vi "Autonomous Independent.vi"() -> ()   [LabVIEW 2015]
doc: "This VI is called when autonomous begins, and will automatically be terminated when autonomous ends. You can carry out timed or sensor driven robot movement independently without needing to return to the caller."
uses:
  <vilib>/Rock Robotics/WPI/RobotDrive/WPI_RobotDriveArcadeDrive_Standard(NoSaturation).vi
  <vilib>/Rock Robotics/Network Tables/NT Read Number.vi
  <vilib>/addons/control/pid/NI_PID_pid.lvlib
  drive/drive.lvclass
  <vilib>/Rock Robotics/Network Tables/NT Write Number.vi
  <vilib>/Rock Robotics/Network Tables/NT Read Boolean.vi
  Robot Global Data.vi
  <vilib>/addons/control/pid/pid.llb/PID (DBL).vi
  <vilib>/Rock Robotics/Network Tables/NT Write Boolean.vi
panel:
  in  "PID turn angle gains":T1={"proportional gain (Kc)"=0.07, "integral time (Ti, min)"=0.0, "derivative time (Td, min)"=1e-05}
  in  "PID arm gains":T1={"proportional gain (Kc)"=1.1, "integral time (Ti, min)"=0.008, "derivative time (Td, min)"=0.0001}
  in  "PID control on":bool
  in  "Angle A?":bool=TRUE
  in  "angle A 2":dbl=30.0
  in  "angle B 2":dbl=90.0
  out "Waveform Chart arm":cluster{"angle B 2":dbl, "Arm Angle":dbl, dbl}(graph)
  in  "Chart slowing 2":i32(knob)=3 scale=1.0..10.0
  in  "Shooter control":dbl(slide) scale=-1.0..1.0
  in  "Arm control":dbl(slide) scale=-1.0..1.0
  in  "Chart slowing":i32(knob)=1 scale=1.0..10.0
  in  "angle B":dbl=90.0
  in  "angle A":dbl
  in  "Reset Gyro":bool
  out "Waveform Chart":cluster{"f":dbl, dbl}(graph)
  in  "Which angle?":bool=TRUE
  out "Stop Wheel Loop":bool
  # "Be sure to right-click and choose Data Operations>>Make Current Value default if you want to save the array values with the VI"
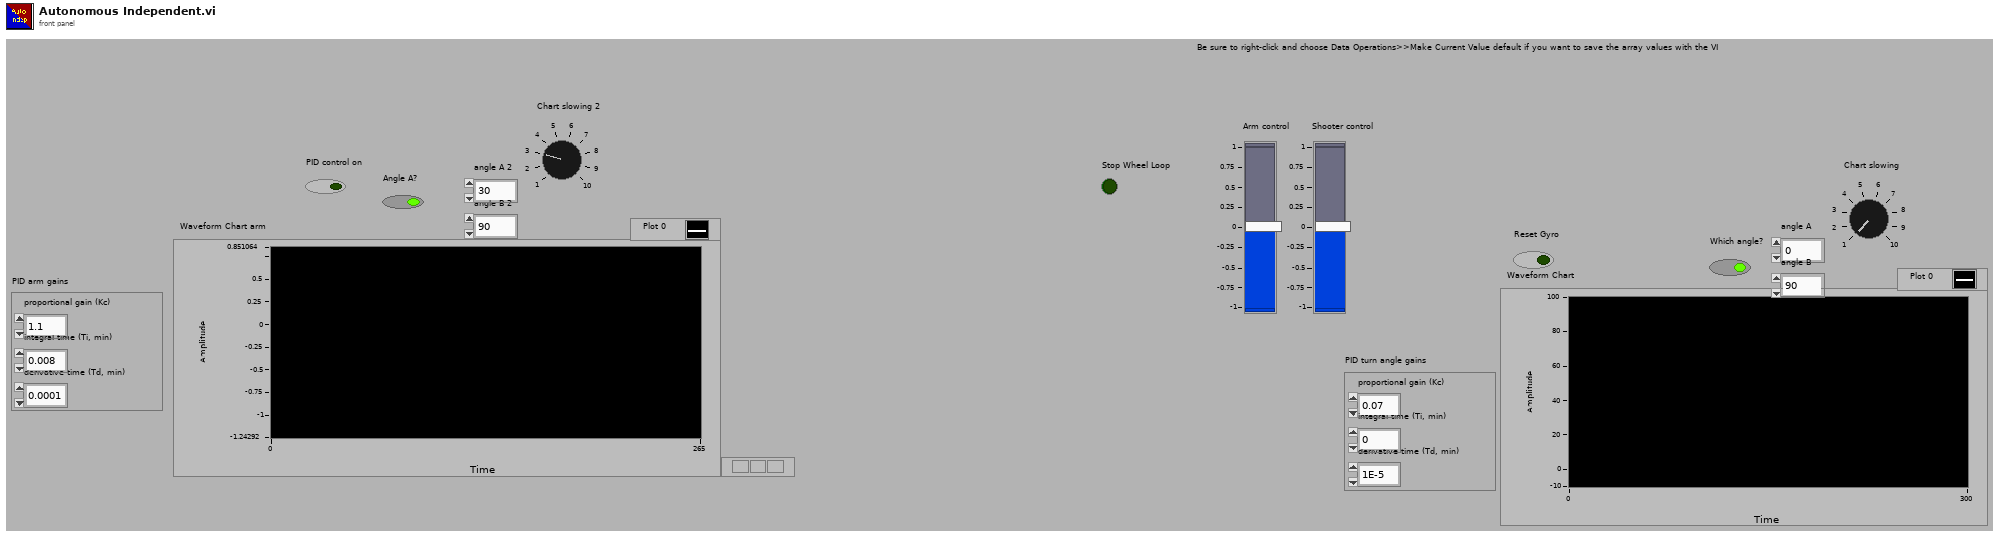
[diagram p1: front panel]
types:
  T1 = cluster{"proportional gain (Kc)":dbl, "integral time (Ti, min)":dbl, "derivative time (Td, min)":dbl}
  T2 = typedef "WPI_GyroDevRef.ctl" = cluster{"DevStatus":errorcluster, "Analog Channel":T3, "Offset":dbl, "Gain (VoltsPerDegree/Second)":dbl, "Gyro Type":enum16{"Analog", "XRS450"}, "Handle":i32, "SPI Bus":T4, "Device Found":bool, "Sample Rate":dbl, "Calibrate On Open":bool}
  T3 = typedef "FPGA_AIChannel.ctl" = enum8{"AI 0", "AI 1", "AI 2", "AI 3", "AI MXP 0", "AI MXP 1", "AI MXP 2", "AI MXP 3", "Invalid"}
  T4 = typedef "spi_bus.ctl" = enum16{"SPI On-Board, CS0", "SPI On-Board, CS1", "SPI On-Board, CS2", "SPI On-Board, CS3", "SPI MXP", "Invalid"}
  T5 = typedef "WPI_PotentiometerDevRef.ctl" = cluster{"DevStatus":errorcluster, "Analog Channel":T3, "Invert Output":bool}
  T6 = typedef "WPI_RobotDriveDevRef.ctl" = cluster{"DevStatus":errorcluster, "Motors[]":T7[], "Square Inputs":bool, "Max Output":dbl}
  T7 = typedef "WPI_MotorControlDeviceRef.ctl" = cluster{"DeviceStatus":errorcluster, "Type":T8, "PWM":cluster{"PWM Channel":T9, "DeadBand":T10}, "CAN":cluster{"Device Number":u8, "Control Mode":T11, "Semaphore":T12, "Max Vout":dbl, "TalonSRX Control Mode":T13}, "Invert":bool}
  T8 = typedef "WPI_MotorControlType.ctl" = enum16{"PWM", "CAN", "CANTalonSRX"}
  T9 = typedef "FPGA_DIOPWMChannel.ctl" = enum8{"PWM 0", "PWM 1", "PWM 2", "PWM 3", "PWM 4", "PWM 5", "PWM 6", "PWM 7", "PWM 8", "PWM 9", "PWM MXP 0", "PWM MXP 1", "PWM MXP 2", "PWM MXP 3", "PWM MXP 4", "PWM MXP 5", "PWM MXP 6", "PWM MXP 7", "PWM MXP 8", "PWM MXP 9", "Invalid"}
  T10 = typedef "WPI_PWMDeadband.ctl" = cluster{"Name":string, "maxPositivePwm":i32, "minPositivePwm":i32, "centerPwm":i32, "maxNegativePwm":i32, "minNegativePwm":i32, "angularRange":u16}
  T11 = typedef "WPI_CANJaguar_ControlMode.ctl" = enum8{"Percent VBus", "Current", "Speed", "Position", "Voltage"}
  T12 = typedef "Semaphore RefNum" = refnum<k1>
  T13 = typedef "WPI_CANTalonSRX_APIControlMode.ctl" = enum8{"Percent VBus", "Speed", "Position", "Slave", "Unchanged / Invalid", "Voltage Compensation", "Current", "Motion Profile"}
  T14 = typedef "WPI_SwitchDevRef.ctl" = cluster{"DevStatus":errorcluster, "DIO Channel":T15, "CntIndex":T16, "Normally Closed":bool}
  T15 = typedef "FPGA_DIOChannel.ctl" = enum8{"DIO 0", "DIO 1", "DIO 2", "DIO 3", "DIO 4", "DIO 5", "DIO 6", "DIO 7", "DIO 8", "DIO 9", "DIO MXP 0", "DIO MXP 1", "DIO MXP 2", "DIO MXP 3", "DIO MXP 4", "DIO MXP 5", "DIO MXP 6", "DIO MXP 7", "DIO MXP 8", "DIO MXP 9", "DIO MXP 10", "DIO MXP 11", "DIO MXP 12", "DIO MXP 13", "DIO MXP 14", "DIO MXP 15", "Invalid"}
  T16 = typedef "FPGA_CounterCtrSystemIndex.ctl" = enum8{"Ctr 0", "Ctr 1", "Ctr 2", "Ctr 3", "Ctr 4", "Ctr 5", "Ctr 6", "Ctr 7", "Invalid"}
  T17 = typedef "WPI_AccelerometerDevRef.ctl" = cluster{"DevStatus":errorcluster, "Scaling":T18, "Analog Channels":T19, "I2C Bus":T20, "SPI Bus":T4, "Accel Range":T21, "ADXL Axes":T22, "Handle":i32, "Device Address":u8, "Accel Type":enum16{"Analog", "ADXL345 I2C", "ADXL345 SPI", "Internal", "ADXL362 SPI"}}
  T18 = typedef "WPI_AccelerometerScaling.ctl" = cluster{"Gain (VoltsPerG)":dbl, "Center Voltage":dbl}
  T19 = typedef "WPI_AccelerometerAnalogChannels.ctl" = cluster{"X-Axis":T3, "Y-Axis":T3, "Z-Axis":T3}
  T20 = typedef "i2c_bus.ctl" = enum16{"I2C On-Board", "I2C MXP", "Invalid"}
  T21 = typedef "ADXL345 Range.ctl" = u8
  T22 = typedef "WPI_AccelerometerADXL345 Axes.ctl" = cluster{"X-Axis":bool, "Y-Axis":bool, "Z-Axis":bool}
  T23 = cluster{"X-Axis":dbl, "Y-Axis":dbl, "Z-Axis":dbl}
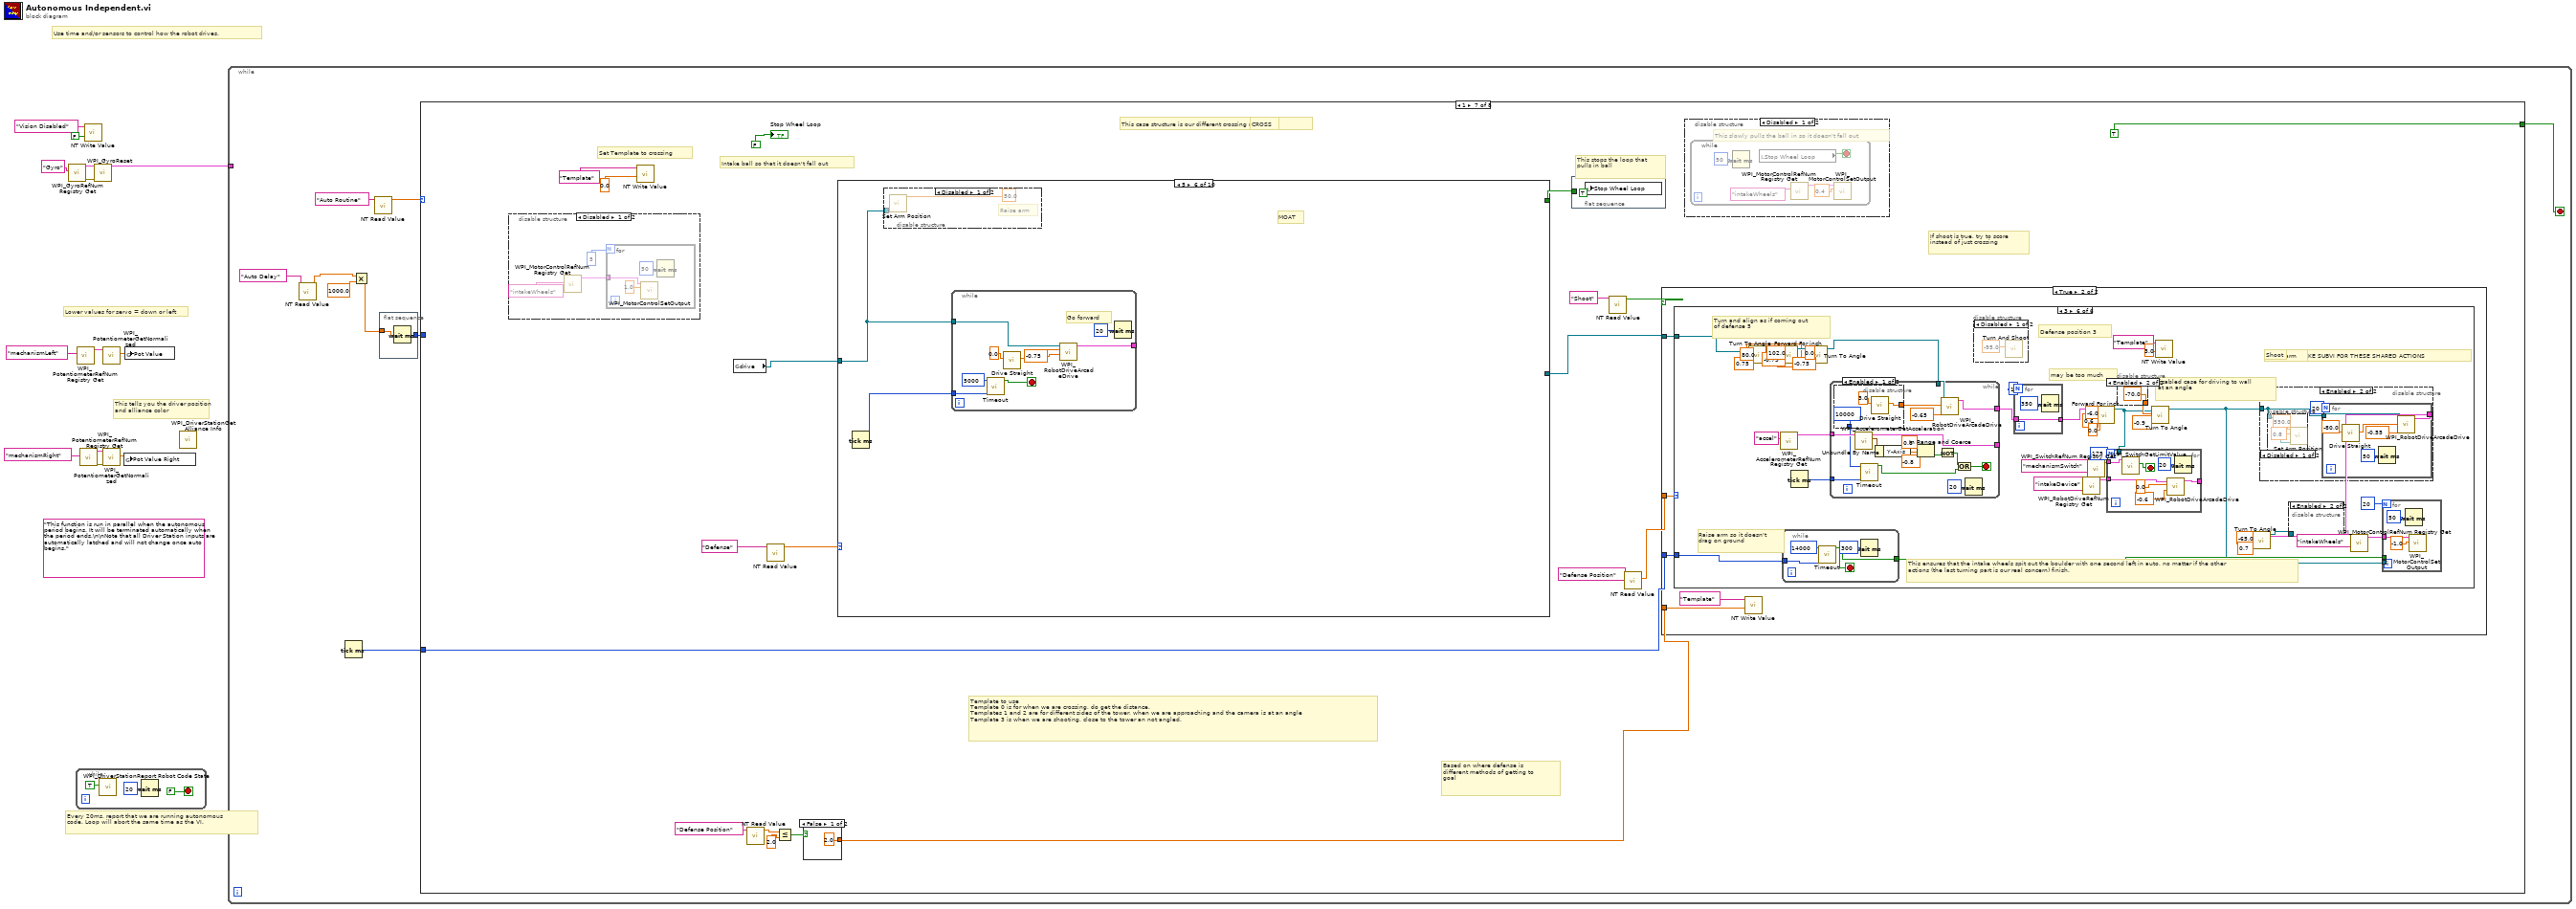
[diagram p0: block diagram]
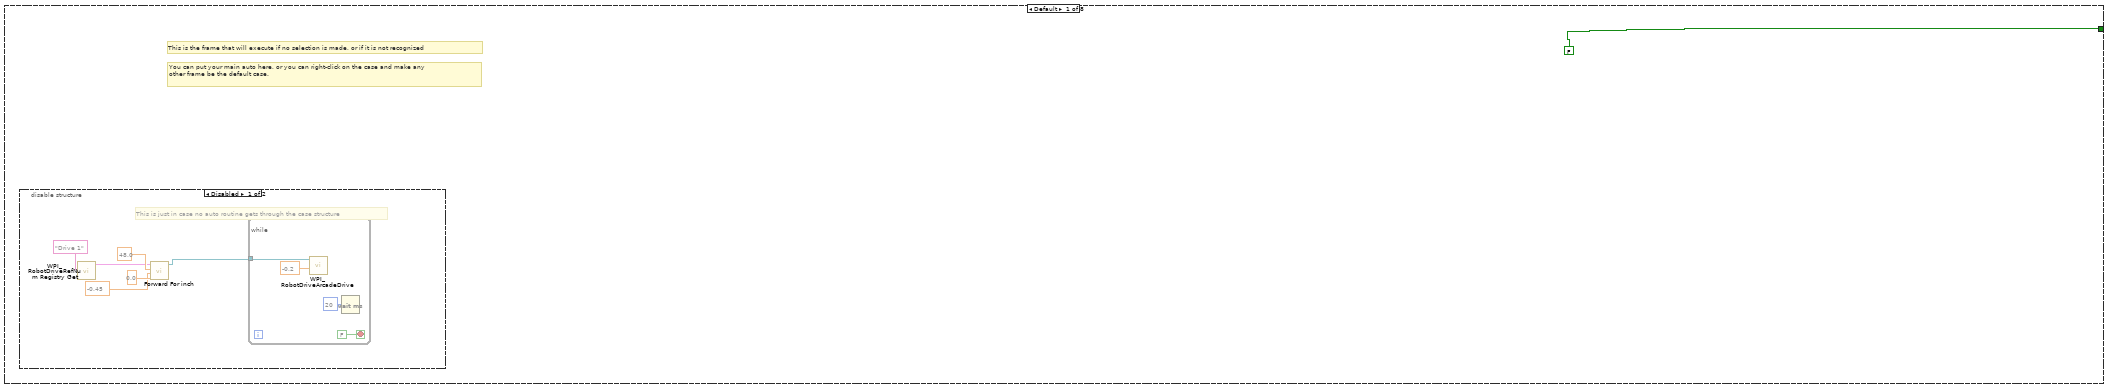
[diagram p2: hidden frame]
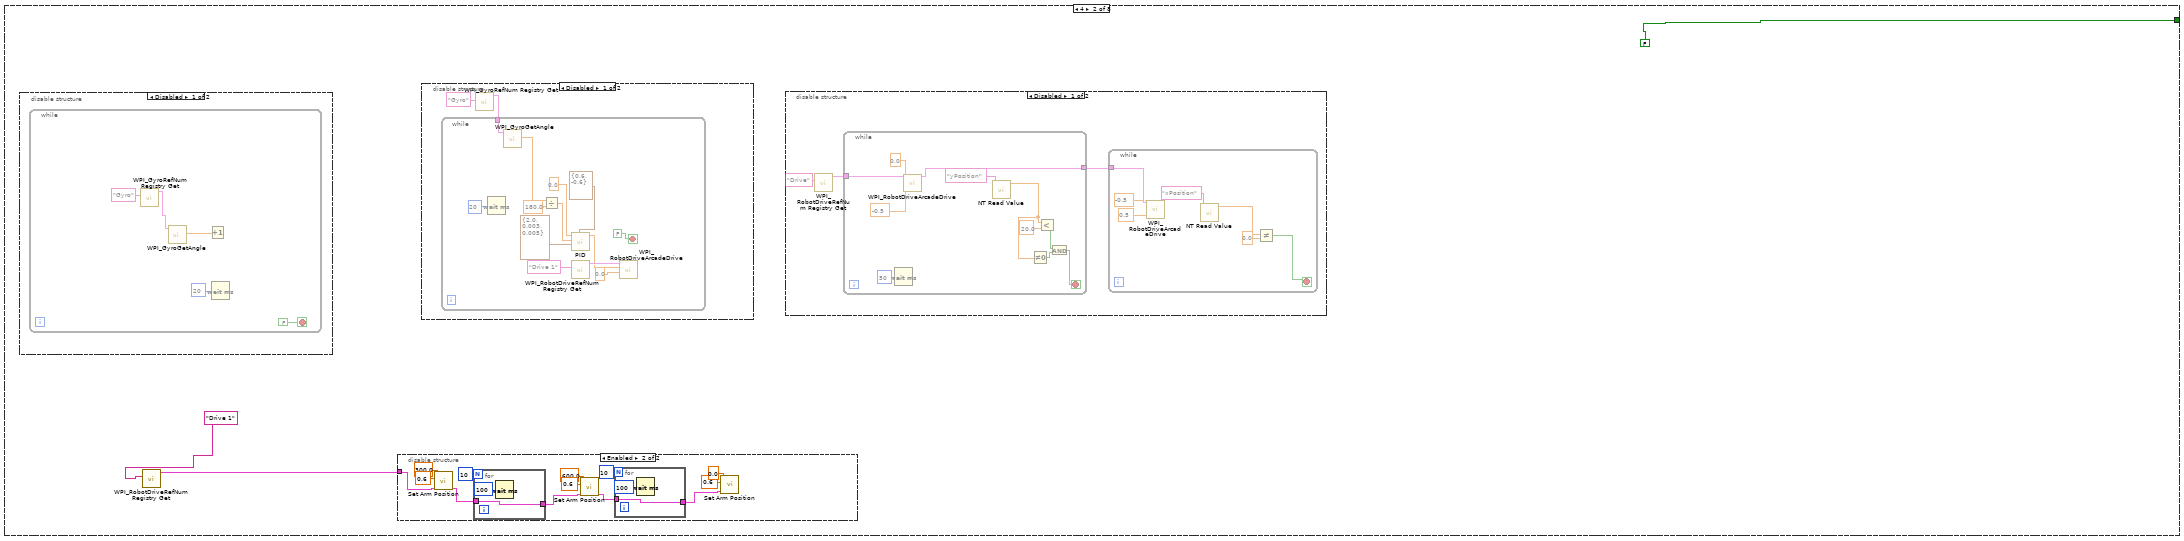
[diagram p4: hidden frame]
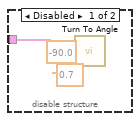
[diagram p5: hidden frame]
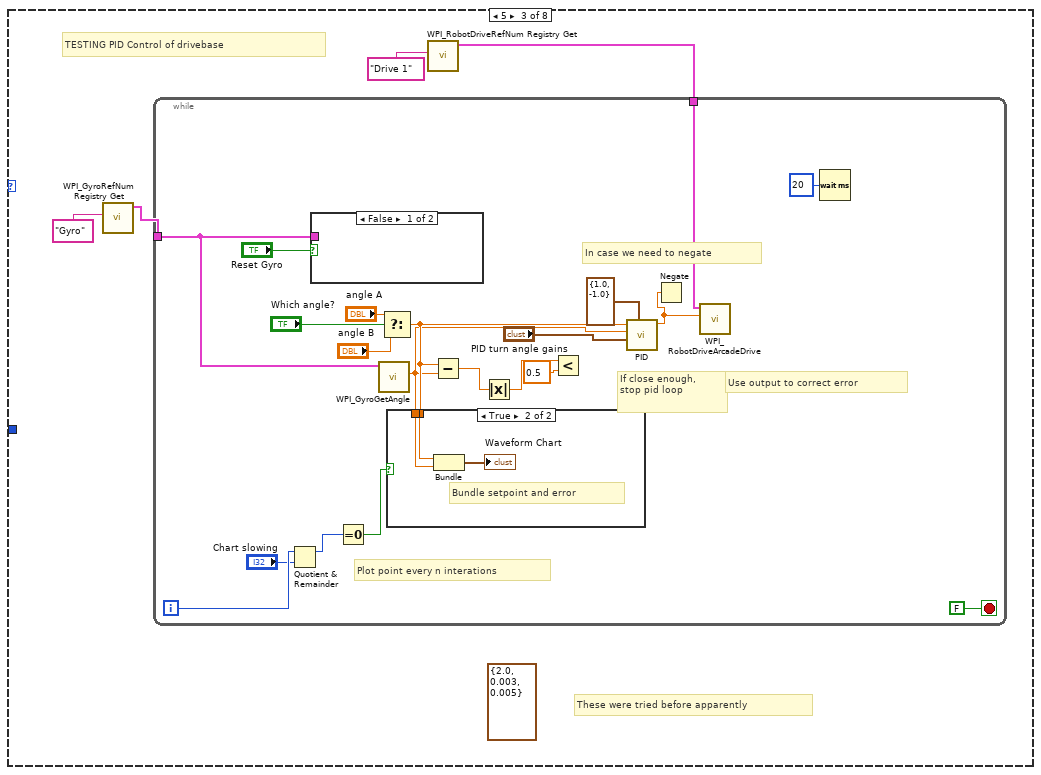
[diagram p9: hidden frame]
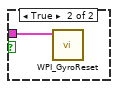
[diagram p11: hidden frame]
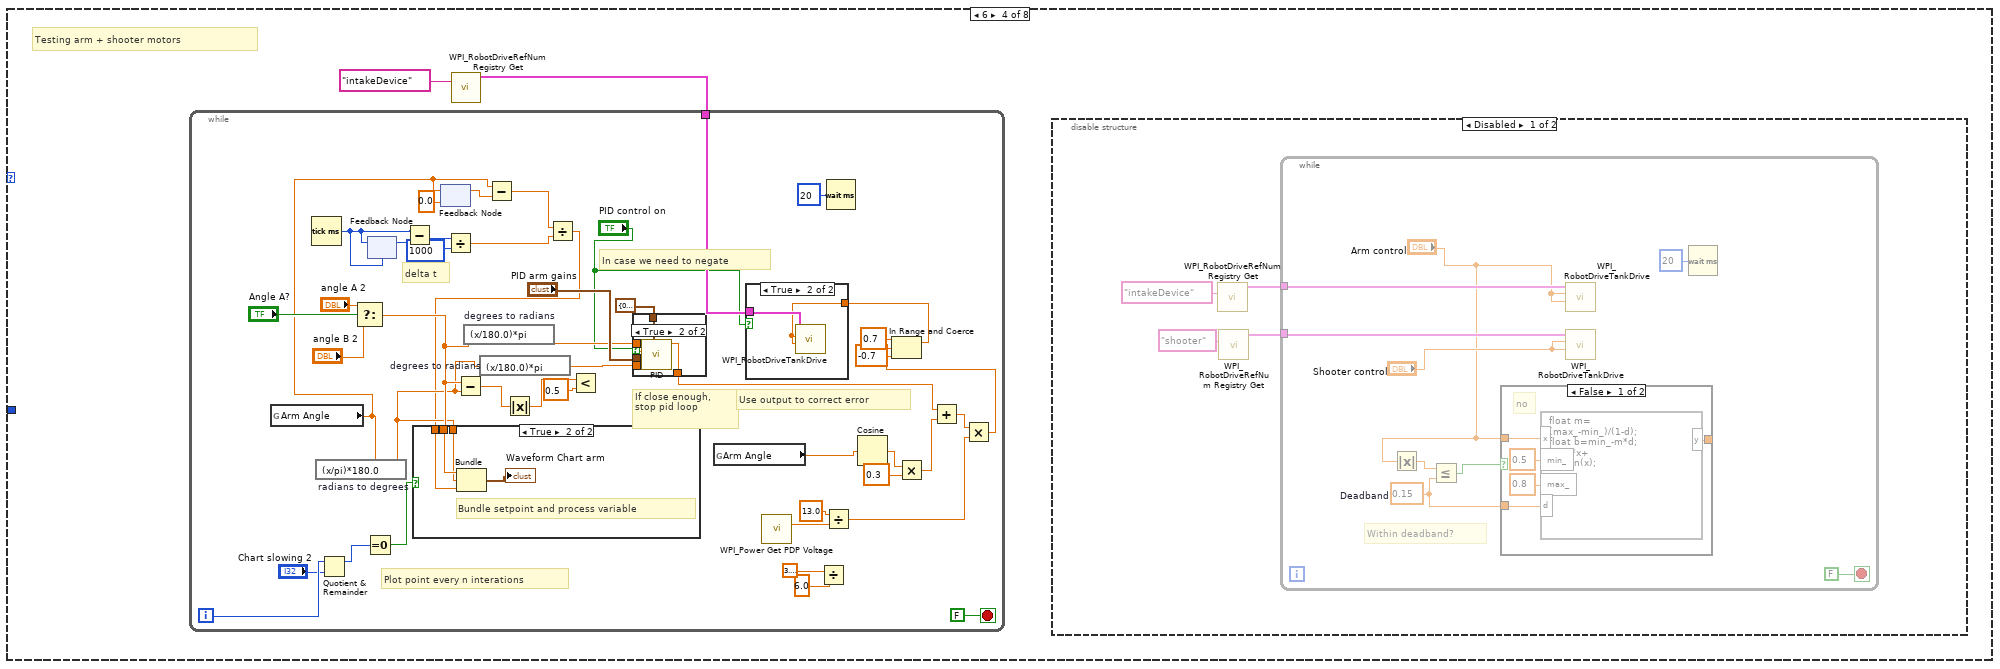
[diagram p12: hidden frame]
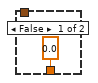
[diagram p14: hidden frame]
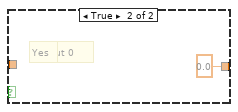
[diagram p16: hidden frame]
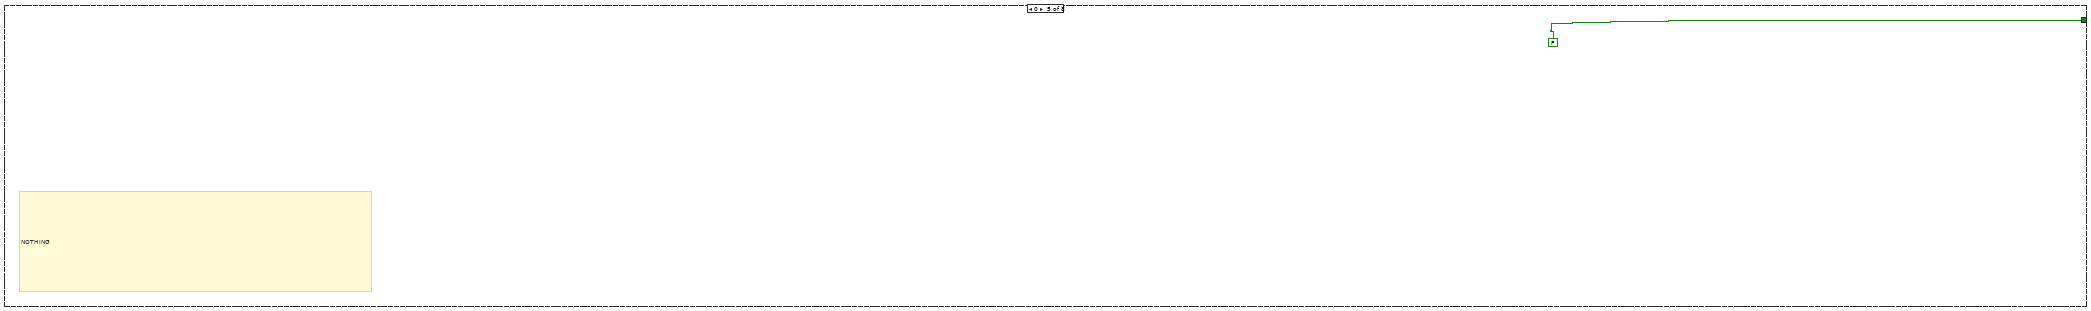
[diagram p18: hidden frame]
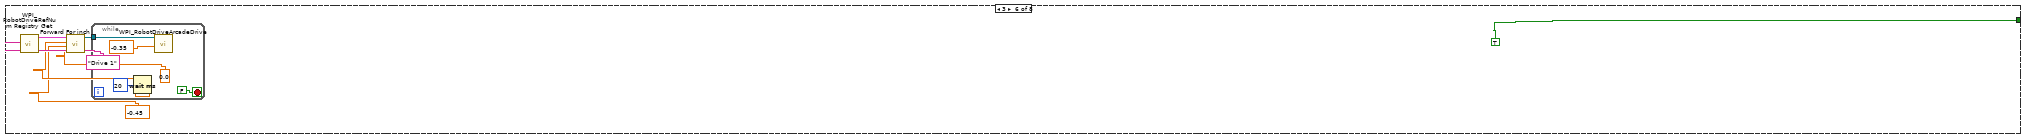
[diagram p19: hidden frame]
diagram:
  (unwired) "This function is run in parallel when the autonomous period begins. It will be terminated automatically when the period ends.\n\nNote that all Driver Station inputs are automatically latched and will not change once auto begins."
  # "Lower values for servo = down or left"
  # "Use time and/or sensors to control how the robot drives."
  # "Every 20ms, report that we are running autonomous\ncode. Loop will abort the same time as the VI."
  # "This tells you the driver position\nand alliance color"
  n1 = call <vilib>:"WPI_GyroRefNum Registry Get.vi"("refnum name"="Gyro") -> ("error out"=w13:errorcluster, "GyroDevRef"=w12:T2)  [unwired: 9 in]
  n2 = while {
    stop <- FALSE stop-if-true
    n3 = call <vilib>:"WPI_DriverStationReport Robot Code State.vi"("Autonomous"=TRUE) -> ()  [unwired: 10 in, 1 out]
    n4 = Wait (ms)(milliseconds to wait=u32 20) -> ()  [unwired: 1 out]
  }
  n5 = call <vilib>:"WPI_PotentiometerRefNum Registry Get.vi"("refnum name"="mechanismLeft") -> ("PotDevRef"=w5:T5)  [unwired: 9 in, 1 out]
  n6 = call <vilib>:"WPI_PotentiometerRefNum Registry Get.vi"("refnum name"="mechanismRight") -> ("error out"=w4:errorcluster, "PotDevRef"=w3:T5)  [unwired: 9 in]
  n7 = call-poly <vilib>:"NT Write Value.vi"("Boolean"=FALSE, "Name"="Vision Disabled") -> ()  [unwired: 9 in, 1 out]
  n8 = call <vilib>:"WPI_GyroReset.vi"("error in"=w13, "GyroDevRef"=w12) -> ("GyroDevRef"=w1:T2)  [unwired: 8 in, 1 out]
  n9 = call <vilib>:"WPI_PotentiometerGetNormalized.vi"("PotDevRef"=w5) -> ("Normalized Value"=w8:dbl)  [unwired: 8 in, 2 out]
  n10 = call <vilib>:"WPI_PotentiometerGetNormalized.vi"("error in"=w4, "PotDevRef"=w3) -> ("Normalized Value"=w2:dbl)  [unwired: 7 in, 2 out]
  n11 = global write "Robot Global Data.vi" "Pot Value Right"(w2) -> ()
  n12 = global write "Robot Global Data.vi" "Pot Value"(w8) -> ()
  n13 = call <vilib>:"WPI_DriverStationGet Alliance Info.vi"() -> ()  [unwired: 12 out]
  n14 = while {
    tunnel: w1 -> [_]
    stop <- w24 stop-if-true
    n15 = call-poly <vilib>:"NT Read Value.vi"("Name"="Auto Delay") -> ("Numeric"=w22:dbl)  [unwired: 9 in, 1 out]
    n16 = Tick Count (ms)() -> (millisecond timer value=w20:u32)
    n17 = Multiply(x=w22, y=1000.0) -> (x*y=w18:dbl)
    n18 = call-poly <vilib>:"NT Read Value.vi"("Name"="Auto Routine") -> ("Numeric"=w19:dbl)  [unwired: 9 in, 1 out]
    n19 = flat-sequence {
      tunnel: w18 -> [w27]
      tunnel: [w26] -> w17
      frame #0 {
        n20 = Wait (ms)(milliseconds to wait=w27) -> (millisecond timer value=w26:u32)
      }
    }
    n21 = case shown="1" w19 {
      tunnel: [FALSE FALSE _ _ FALSE TRUE TRUE TRUE] -> w24
      tunnel: w20 -> [_ _ _ _ _ _ w223 _]
      tunnel: w17 -> [_ _ _ _ _ _ _ _]
      frame Default {
        # "You can put your main auto here, or you can right-click on the case and make any\nother frame be the default case."
        # "This is the frame that will execute if no selection is made, or if it is not recognized"
        n22 = disable-structure shown="Disabled" {
          frame Disabled {
            # "This is just in case no auto routine gets through the case structure"
            n23 = call <vilib>:"WPI_RobotDriveRefNum Registry Get.vi"("refnum name"="Drive 1") -> ("RobotDriveDevRef"=w30:T6)  [unwired: 9 in, 1 out]
            n24 = call "Forward For inch.vi"("Angle"=0.0 ("Angle robot facing"), "Speed"=-0.45, "Distance"=48.0, "drive.lvclass"=w30) -> ("drive.lvclass"=w34:refnum<class "drive.lvclass">)  [unwired: 7 in]
            n25 = while {
              tunnel: w34 -> [w36]
              stop <- FALSE stop-if-true
              n26 = call-poly <vilib>:"WPI_RobotDriveArcadeDrive.vi"("Y axis value"=-0.2, "RobotDriveDevRef"=w36) -> ()  [unwired: 7 in, 3 out]
              n27 = Wait (ms)(milliseconds to wait=u32 20) -> ()  [unwired: 1 out]
            }
          }
          frame Enabled {
          }
        }
      }
      frame 4 {
        n28 = disable-structure shown="Disabled" {
          frame Disabled {
            n29 = while {
              stop <- FALSE stop-if-true
              n30 = call <vilib>:"WPI_GyroRefNum Registry Get.vi"("refnum name"="Gyro") -> ("GyroDevRef"=w63:T2)  [unwired: 9 in, 1 out]
              n31 = call <vilib>:"WPI_GyroGetAngle.vi"("GyroDevRef"=w63) -> ("Angle"=w64:dbl)  [unwired: 6 in, 4 out]
              n32 = Increment(x=w64) -> ()  [unwired: 1 out]
              n33 = Wait (ms)(milliseconds to wait=u32 20) -> ()  [unwired: 1 out]
            }
          }
          frame Enabled {
          }
        }
        n34 = call <vilib>:"WPI_RobotDriveRefNum Registry Get.vi"("refnum name"="Drive 1") -> ("RobotDriveDevRef"=w39:T6)  [unwired: 9 in, 1 out]
        n35 = disable-structure shown="Enabled" {
          disable-tunnel: w39 -> [w42 w57]
          frame Disabled {
            n36 = call "Turn To Angle.vi"(7:w42, "Speed/Direction"=0.7, "Angle"=-90.0) -> ()  [unwired: 8 in, 1 out]
          }
          frame Enabled {
            n37 = call "Set Arm Position.vi"("RobotDriveDevRef 2"=w57, "Speed"=0.6, "Setpoint"=300.0) -> ("RobotDriveDevRef"=w50:T6)  [unwired: 8 in]
            n38 = for {
              N: 10 -> [_]
              tunnel: [w60] -> w51
              tunnel: w50 -> [w60]
              n39 = Wait (ms)(milliseconds to wait=u32 100) -> ()  [unwired: 1 out]
            }
            n40 = call "Set Arm Position.vi"("RobotDriveDevRef 2"=w51, "Speed"=0.6, "Setpoint"=600.0) -> ("RobotDriveDevRef"=w45:T6)  [unwired: 8 in]
            n41 = for {
              N: 10 -> [_]
              tunnel: [w58] -> w46
              tunnel: w45 -> [w58]
              n42 = Wait (ms)(milliseconds to wait=u32 100) -> ()  [unwired: 1 out]
            }
            n43 = call "Set Arm Position.vi"("RobotDriveDevRef 2"=w46, "Speed"=0.6, "Setpoint"=0.0) -> ()  [unwired: 8 in, 1 out]
          }
        }
        n44 = disable-structure shown="Disabled" {
          frame Disabled {
            n45 = call <vilib>:"WPI_GyroRefNum Registry Get.vi"("refnum name"="Gyro") -> ("GyroDevRef"=w88:T2)  [unwired: 9 in, 1 out]
            n46 = while {
              tunnel: w88 -> [w99]
              stop <- FALSE stop-if-true
              n47 = Wait (ms)(milliseconds to wait=u32 20) -> ()  [unwired: 1 out]
              n48 = call <vilib>:"WPI_GyroGetAngle.vi"("GyroDevRef"=w99) -> ("Angle"=w101:dbl)  [unwired: 6 in, 4 out]
              n49 = Divide(x=w101, y=180.0) -> (x/y=w91:dbl)
              n50 = call-poly <vilib>:"PID.vi"("output range"=cluster{"output high":dbl, "output low":dbl} {"output high"=0.6, "output low"=-0.6}, "PID gains"=T1 {"proportional gain (Kc)"=2.0, "integral time (Ti, min)"=0.003, "derivative time (Td, min)"=0.005} ("Drive straight"), "process variable"=w91, "setpoint"=0.0) -> ("output"=w90:dbl)  [unwired: 6 in, 1 out]
              n51 = call <vilib>:"WPI_RobotDriveRefNum Registry Get.vi"("refnum name"="Drive 1") -> ("RobotDriveDevRef"=w97:T6)  [unwired: 1 in, 9 out]
              n52 = call-poly <vilib>:"WPI_RobotDriveArcadeDrive.vi"("Y axis value"=0.0, "X axis value"=w90, "RobotDriveDevRef"=w97) -> ()  [unwired: 6 in, 3 out]
            }
          }
          frame Enabled {
          }
        }
        n53 = disable-structure shown="Disabled" {
          frame Disabled {
            n54 = call <vilib>:"WPI_RobotDriveRefNum Registry Get.vi"("refnum name"="Drive") -> ("RobotDriveDevRef"=w68:T6)  [unwired: 9 in, 1 out]
            n55 = while {
              tunnel: w68 -> [w84]
              tunnel: [w82] -> w67
              stop <- w77 stop-if-true
              n56 = Wait (ms)(milliseconds to wait=u32 50) -> ()  [unwired: 1 out]
              n57 = call-poly <vilib>:"WPI_RobotDriveArcadeDrive.vi"("Y axis value"=-0.5, "X axis value"=0.0, "RobotDriveDevRef"=w84) -> ("RobotDriveDevRef"=w82:T6)  [unwired: 6 in, 2 out]
              n58 = call-poly <vilib>:"NT Read Value.vi"("Name"="yPosition") -> ("Numeric"=w79:dbl)  [unwired: 9 in, 1 out]
              n59 = Not Equal To 0?(x=w79) -> (x != 0?=w78:bool)
              n60 = Less?(x=w79, y=20.0) -> (x < y?=w80:bool)
              n61 = And(x=w80, y=w78) -> (x .and. y?=w77:bool)
            }
            n62 = while {
              tunnel: w67 -> [w76]
              stop <- w72 stop-if-true
              n63 = call-poly <vilib>:"WPI_RobotDriveArcadeDrive.vi"("Y axis value"=0.5, "X axis value"=-0.5, "RobotDriveDevRef"=w76) -> ()  [unwired: 6 in, 3 out]
              n64 = call-poly <vilib>:"NT Read Value.vi"("Name"="xPosition") -> ("Numeric"=w74:dbl)  [unwired: 9 in, 1 out]
              n65 = Not Equal?(x=w74, y=0.0) -> (x != y?=w72:bool)
            }
          }
          frame Enabled {
          }
        }
      }
      frame 5 {
        (unwired) T1 {"proportional gain (Kc)"=2.0, "integral time (Ti, min)"=0.003, "derivative time (Td, min)"=0.005} ("Drive straight")
        # "These were tried before apparently"
        # "TESTING PID Control of drivebase"
        n66 = call <vilib>:"WPI_GyroRefNum Registry Get.vi"("refnum name"="Gyro") -> ("GyroDevRef"=w106:T2)  [unwired: 9 in, 1 out]
        n67 = call <vilib>:"WPI_RobotDriveRefNum Registry Get.vi"("refnum name"="Drive 1") -> ("RobotDriveDevRef"=w103:T6)  [unwired: 9 in, 1 out]
        n68 = while {
          tunnel: w106 -> [w110]
          tunnel: w103 -> [w109]
          i -> [w112]
          stop <- FALSE stop-if-true
          # "In case we need to negate"
          # "Plot point every n interations"
          # "If close enough,\nstop pid loop"
          # "Use output to correct error"
          n69 = Quotient & Remainder(x=w112, y="Chart slowing") -> (x-y*floor(x/y)=w114:i32)  [unwired: 1 out]
          n70 = case shown="False" "Reset Gyro" {
            tunnel: w110 -> [_ w130]
            frame False {
            }
            frame True {
              n71 = call <vilib>:"WPI_GyroReset.vi"("GyroDevRef"=w130) -> ()  [unwired: 9 in, 2 out]
            }
          }
          n72 = Equal To 0?(x=w114) -> (x = 0?=w113:bool)
          n73 = call <vilib>:"WPI_GyroGetAngle.vi"("GyroDevRef"=w110) -> ("Angle"=w122:dbl)  [unwired: 6 in, 4 out]
          n74 = Select(t="angle A", s="Which angle?", f="angle B") -> (s? t:f=w124:dbl)
          n75 = case shown="True" w113 {
            tunnel: w124 -> [_ w128]
            tunnel: w122 -> [_ w127]
            frame False {
            }
            frame True {
              # "Bundle setpoint and error"
              n76 = Bundle("angle B"=w128, "Angle"=w127) -> (→"Waveform Chart":cluster{"angle B":dbl, "Angle":dbl})  [unwired: 1 in]
            }
          }
          n77 = Subtract(x=w124, y=w122) -> (x-y=w120:dbl)
          n78 = Absolute Value(x=w120) -> (abs(x)=w119:dbl)
          n79 = Less?(x=w119, y=0.5) -> ()  [unwired: 1 out]
          n80 = call-poly <vilib>:"PID.vi"("output range"=cluster{"output high":dbl, "output low":dbl} {"output high"=1.0, "output low"=-1.0}, "PID gains"="PID turn angle gains", "process variable"=w122, "setpoint"=w124) -> ("output"=w108:dbl)  [unwired: 6 in, 1 out]
          n81 = Negate(x=w108) -> ()  [unwired: 1 out]
          n82 = call-poly <vilib>:"WPI_RobotDriveArcadeDrive.vi"("X axis value"=w108, "RobotDriveDevRef"=w109) -> ()  [unwired: 7 in, 3 out]
          n83 = Wait (ms)(milliseconds to wait=u32 20) -> ()  [unwired: 1 out]
        }
      }
      frame 6 {
        # "Testing arm + shooter motors"
        n84 = call <vilib>:"WPI_RobotDriveRefNum Registry Get.vi"("refnum name"="intakeDevice") -> ("RobotDriveDevRef"=w132:T6)  [unwired: 9 in, 1 out]
        n85 = while {
          tunnel: w132 -> [w164]
          i -> [w166]
          stop <- FALSE stop-if-true
          # "delta t"
          # "In case we need to negate"
          # "Plot point every n interations"
          # "If close enough,\nstop pid loop"
          # "Use output to correct error"
          n86 = global read "Robot Global Data.vi" "Arm Angle"() -> (w134:dbl)
          n87 = Tick Count (ms)() -> (millisecond timer value=w141:u32)
          n88 = expression code="(x/pi)*180.0" "radians to degrees"(w134) -> (w143:dbl)
          n89 = Quotient & Remainder(x=w166, y="Chart slowing 2") -> (x-y*floor(x/y)=w168:i32)  [unwired: 1 out]
          n90 = Select(t="angle A 2", s="Angle A?", f="angle B 2") -> (s? t:f=w158:dbl)
          n91 = Equal To 0?(x=w168) -> (x = 0?=w167:bool)
          n92 = feedback #1(w141) -> (w142:u32)
          n93 = feedback-in #1(w141) -> ()
          n94 = Subtract(x=w141, y=w142) -> (x-y=w140:u32)
          n95 = feedback #2(0.0 ("Arm Angle")) -> (w138:dbl)
          n96 = feedback-in #2(w134) -> ()
          n97 = Divide(x=w140, y=u32 1000) -> (x/y=w135:dbl)
          n98 = Subtract(x=w158, y=w143) -> (x-y=w157:dbl)
          n99 = expression code="(x/180.0)*pi" "degrees to radians"(w158) -> (w159:dbl)
          n100 = expression code="(x/180.0)*pi" "degrees to radians"(w143) -> (w146:dbl)
          n101 = Subtract(x=w134, y=w138) -> (x-y=w136:dbl)
          n102 = Absolute Value(x=w157) -> (abs(x)=w173:dbl)
          n103 = Divide(x=w136, y=w135) -> (x/y=w133:dbl)
          n104 = case shown="True" w167 {
            tunnel: w158 -> [_ w189]
            tunnel: w143 -> [_ w188]
            tunnel: w133 -> [_ w186]
            frame False {
            }
            frame True {
              # "Bundle setpoint and process variable"
              n105 = Bundle("angle B 2"=w189, "Arm Angle"=w188, w186) -> (→"Waveform Chart arm":cluster{"angle B 2":dbl, "Arm Angle":dbl, dbl})  [unwired: 1 in]
            }
          }
          n106 = Less?(x=w173, y=0.5) -> ()  [unwired: 1 out]
          n107 = case shown="True" "PID control on" {
            tunnel: "PID arm gains" -> [_ w185]
            tunnel: cluster{"output high":dbl, "output low":dbl} {"output high"=0.7, "output low"=-0.7} ("output range") -> [_ w184]
            tunnel: w159 -> [_ w183]
            tunnel: w146 -> [_ w182]
            tunnel: [0.0 ("output") w181] -> w145
            frame False {
            }
            frame True {
              n108 = call-poly <vilib>:"PID.vi"("output range"=w184, "PID gains"=w185, "process variable"=w182, "setpoint"=w183) -> ("output"=w181:dbl)  [unwired: 6 in, 1 out]
            }
          }
          n109 = global read "Robot Global Data.vi" "Arm Angle"() -> (w153:dbl)
          n110 = call <vilib>:"WPI_Power Get PDP Voltage.vi"() -> ("voltage (V)"=w163:dbl)  [unwired: 14 in, 1 out]
          n111 = Divide(x=3.141592653589793, y=6.0) -> ()  [unwired: 1 out]
          n112 = Divide(x=13.0, y=w163) -> (x/y=w151:dbl)
          n113 = Wait (ms)(milliseconds to wait=u32 20) -> ()  [unwired: 1 out]
          n114 = Cosine(x=w153) -> (cos(x)=w156:dbl)
          n115 = Multiply(x=w156, y=0.3) -> (x*y=w154:dbl)
          n116 = Add(x=w145, y=w154) -> (x+y=w152:dbl)
          n117 = Multiply(x=w152, y=w151) -> (x*y=w150:dbl)
          n118 = In Range and Coerce(upper limit=0.7, x=w150, lower limit=-0.7) -> (coerced(x)=w147:dbl)  [unwired: 1 out]
          n119 = case shown="True" "PID control on" {
            tunnel: w164 -> [_ w179]
            tunnel: w147 -> [_ w178]
            frame False {
            }
            frame True {
              n120 = call <vilib>:"WPI_RobotDriveTankDrive.vi"("Right axis value"=w178, "Left axis value"=w178, "RobotDriveDevRef"=w179) -> ()  [unwired: 6 in, 3 out]
            }
          }
        }
        n121 = disable-structure shown="Disabled" {
          frame Disabled {
            n122 = call <vilib>:"WPI_RobotDriveRefNum Registry Get.vi"("refnum name"="intakeDevice") -> ("RobotDriveDevRef"=w193:T6)  [unwired: 9 in, 1 out]
            n123 = call <vilib>:"WPI_RobotDriveRefNum Registry Get.vi"("refnum name"="shooter") -> ("RobotDriveDevRef"=w192:T6)  [unwired: 9 in, 1 out]
            n124 = while {
              tunnel: w193 -> [w201]
              tunnel: w192 -> [w200]
              stop <- FALSE stop-if-true
              w196 = 0.15  # Deadband
              # "Within deadband?"
              n125 = Absolute Value(x="Arm control") -> (abs(x)=w198:dbl)
              n126 = Less Or Equal?(x=w198, y=w196) -> (x <= y?=w197:bool)
              n127 = case shown="False" w197 {
                tunnel: [w207 0.0 ("y")] -> _
                tunnel: "Arm control" -> [w204 _]
                tunnel: w196 -> [w203 _]
                frame False {
                  # "no"
                  n128 = formula code="float m= \n(max_-min_)/(1-d);\nfloat b=min_-m*d;\ny=m*x+\nb*sign(x);"("x"=w204, "min_"=0.5 ("input variable"), "max_"=0.8 ("input variable"), "d"=w203) -> ("y"=w207:dbl)
                }
                frame True {
                  # "Yes"
                  # "Output 0"
                }
              }
              n129 = call <vilib>:"WPI_RobotDriveTankDrive.vi"("Right axis value"="Arm control", "Left axis value"="Arm control", "RobotDriveDevRef"=w201) -> ()  [unwired: 6 in, 3 out]
              n130 = call <vilib>:"WPI_RobotDriveTankDrive.vi"("Right axis value"="Shooter control", "Left axis value"="Shooter control", "RobotDriveDevRef"=w200) -> ()  [unwired: 6 in, 3 out]
              n131 = Wait (ms)(milliseconds to wait=u32 20) -> ()  [unwired: 1 out]
            }
          }
          frame Enabled {
          }
        }
      }
      frame 0 {
        # "NOTHING"
      }
      frame 3 {
        n132 = call <vilib>:"WPI_RobotDriveRefNum Registry Get.vi"("refnum name"="Drive 1") -> ("RobotDriveDevRef"=w215:T6)  [unwired: 9 in, 1 out]
        n133 = call "Forward For inch.vi"("Angle"=0.0 ("Angle robot facing"), "Speed"=-0.45, "Distance"=48.0, "drive.lvclass"=w215) -> ("drive.lvclass"=w211:refnum<class "drive.lvclass">)  [unwired: 7 in]
        n134 = while {
          tunnel: w211 -> [w218]
          stop <- FALSE stop-if-true
          n135 = Wait (ms)(milliseconds to wait=u32 20) -> ()  [unwired: 1 out]
          n136 = call-poly <vilib>:"WPI_RobotDriveArcadeDrive.vi"("Y axis value"=-0.35, "RobotDriveDevRef"=w218) -> ()  [unwired: 7 in, 3 out]
        }
      }
      frame 1 {
        # "CROSS"
        # "This stops the loop that\npulls in ball"
        # "Based on where defense is\ndifferent methods of getting to\ngoal"
        # "If shoot is true, try to score\ninstead of just crossing"
        # "This case structure is our different crossing methods"
        # "Intake ball so that it doesn't fall out"
        # "Set Template to crossing"
        # "Template to use\nTemplate 0 is for when we are crossing, do get the distance.\nTemplates 1 and 2 are for different sides of the tower, when we are approaching and the camera is at an angle\nTemplate 3 is when we are shooting, close to the tower an not angled."
        n137 = disable-structure shown="Disabled" {
          frame Disabled {
            n138 = call <vilib>:"WPI_MotorControlRefNum Registry Get.vi"("refnum name"="intakeWheels") -> ("MotorControlDevRef"=w245:T7)  [unwired: 9 in, 1 out]
            n139 = for {
              N: 5 -> [_]
              tunnel: w245 -> [w248]
              n140 = call <vilib>:"WPI_MotorControlSetOutput.vi"("Output"=1.0, "MotorControlDevRef"=w248) -> ()  [unwired: 7 in, 3 out]
              n141 = Wait (ms)(milliseconds to wait=u32 50) -> ()  [unwired: 1 out]
            }
          }
          frame Enabled {
          }
        }
        n142 = call-poly <vilib>:"NT Write Value.vi"("Numeric"=0.0, "Name"="Template") -> ()  [unwired: 9 in, 1 out]
        n143 = global read "Robot Global Data.vi" "drive"() -> (w222:refnum<class "drive.lvclass">)
        n144 = call-poly <vilib>:"NT Read Value.vi"("Name"="Defense Position") -> ("Numeric"=w229:dbl)  [unwired: 9 in, 1 out]
        n145 = call-poly <vilib>:"NT Read Value.vi"("Name"="Defense") -> ("Numeric"=w237:dbl)  [unwired: 9 in, 1 out]
        n146 = Less Or Equal?(x=w229, y=2.0) -> (x <= y?=w231:bool)
        n147 = case shown="False" w231 {
          tunnel: [2.0 ("Speed/Direction") 1.0 ("Speed/Direction")] -> w227
          frame False {
          }
          frame True {
          }
        }
        n148 = case shown="5" w237 {
          tunnel: w222 -> [w254 w266 w286 w411 w494 w511 w525 w536 w551 w566]
          tunnel: [FALSE _ _ _ _ _ _ _ _ _] -> w233
          tunnel: [_ w256 _ _ _ _ _ _ _ _] -> w221
          frame 0, Default {
          }
          frame 1 {
            # "If we decide to drive to castle wall at an angle,\nthe code in the enabled structure will be disabled\nand code will be enabled in the next case structure\nit drive at an angle"
            # "Lower arm"
            # "Go under bar, up to align with low goal"
            # "Go forward fast (to save time)"
            # "Pause"
            # "LOW BAR"
            n149 = call <vilib>:"WPI_SwitchRefNum Registry Get.vi"("refnum name"="mechanismSwitch") -> ("SwitchDevRef"=w259:T14)  [unwired: 9 in, 1 out]
            n150 = call <vilib>:"WPI_RobotDriveRefNum Registry Get.vi"("refnum name"="intakeDevice") -> ("RobotDriveDevRef"=w258:T6)  [unwired: 9 in, 1 out]
            n151 = for {
              N: 1 -> [_]
              tunnel: [w284] -> w257
              tunnel: w266 -> [w284]
              n152 = Wait (ms)(milliseconds to wait=u32 350) -> ()  [unwired: 1 out]
            }
            n153 = disable-structure shown="Enabled" {
              disable-tunnel: w266 -> [w276 _]
              disable-tunnel: w259 -> [_ w278]
              disable-tunnel: w258 -> [_ w277]
              frame Disabled {
                n154 = call "Set Arm Position.vi"("RobotDriveDevRef 2"=w276, "Speed"=0.95, "Setpoint"=510.0) -> ()  [unwired: 8 in, 1 out]
              }
              frame Enabled {
                n155 = while {
                  tunnel: w278 -> [w280]
                  tunnel: w277 -> [w279]
                  stop <- w281 stop-if-true
                  n156 = call <vilib>:"WPI_SwitchGetLimitValue.vi"("SwitchDevRef"=w280) -> ("Switch Pressed"=w281:bool)  [unwired: 8 in, 2 out]
                  n157 = call-poly <vilib>:"WPI_RobotDriveArcadeDrive.vi"("Y axis value"=-0.7, "X axis value"=0.0, "RobotDriveDevRef"=w279) -> ()  [unwired: 6 in, 3 out]
                }
              }
            }
            n158 = call "Forward For Inch.vi"("Angle"=0.0 ("Angle robot facing"), "Speed"=0.78, "Distance"=-32.0, "drive.lvclass"=w257) -> ("drive.lvclass"=w262:refnum<class "drive.lvclass">)  [unwired: 7 in]
            n159 = disable-structure shown="Enabled" {
              disable-tunnel: [w269 w273] -> w256
              disable-tunnel: w262 -> [w268 w273]
              frame Enabled {
                n160 = call "Forward For Inch.vi"("Angle"=5.0 ("Angle robot facing"), "Speed"=0.67, "Distance"=-172.0, "drive.lvclass"=w268) -> ("drive.lvclass"=w269:refnum<class "drive.lvclass">)  [unwired: 7 in]
              }
              frame Disabled {
              }
            }
          }
          frame 2 {
            # "PORTCULLIS"
            n161 = disable-structure shown="Enabled" {
              disable-tunnel: [w298 w360] -> w287
              disable-tunnel: w286 -> [w290 w375]
              frame Disabled {
                # "then pause while arm\nlowering"
                # "Pause"
                # "Because we had trouble making it go far\nenough, add a burst of movement at the end"
                # "We think the arm wasn't rasing\nbecause forward for inch wasn't\nending, so we added a time value instead"
                # "I'M SORRY THS IS SO COMPLICATED"
                # "Go forward slowly, so we \ndon't roll off ramp. When arm is high \nenough, start moving forward"
                # "raise arm, and porticullis"
                # "pause"
                # "Go forward to\nporticullus"
                # "Lower arm"
                n162 = for {
                  N: 1 -> [_]
                  tunnel: w290 -> [w355]
                  tunnel: [w355] -> w302
                  n163 = Wait (ms)(milliseconds to wait=u32 750) -> ()  [unwired: 1 out]
                }
                n164 = call "Set Arm Position.vi"("RobotDriveDevRef 2"=w290, "Speed"=0.7, "Setpoint"=700.0) -> ()  [unwired: 8 in, 1 out]
                n165 = global read "Robot Global Data.vi" "Pot Value"() -> (w294:dbl)
                n166 = call <vilib>:"WPI_PotentiometerRefNum Registry Get.vi"("refnum name"="mechanismLeft") -> ("PotDevRef"=w295:T5)  [unwired: 9 in, 1 out]
                n167 = call "Forward For inch.vi"("Angle"=0.0 ("Angle robot facing"), "Speed"=-0.5, "Distance"=47.0, "drive.lvclass"=w302) -> ("drive.lvclass"=w305:refnum<class "drive.lvclass">)  [unwired: 7 in]
                n168 = call <vilib>:"WPI_RobotDriveRefNum Registry Get.vi"("refnum name"="Drive 1") -> ("RobotDriveDevRef"=w299:T6)  [unwired: 9 in, 1 out]
                n169 = flat-sequence {
                  tunnel: [w310] -> w297
                  tunnel: w291 -> [_]
                  frame #0 {
                    n170 = Tick Count (ms)() -> (millisecond timer value=w310:u32)
                  }
                }
                n171 = for {
                  N: 1 -> [_]
                  tunnel: w305 -> [w357]
                  tunnel: [w357] -> w291
                  n172 = Wait (ms)(milliseconds to wait=u32 200) -> ()  [unwired: 1 out]
                }
                n173 = while {
                  tunnel: w297 -> [w338]
                  tunnel: w291 -> [w333]
                  tunnel: [w332] -> w292
                  stop <- w336 stop-if-true
                  n174 = call "Timeout.vi"("Start Time In"=w338, "Time Limit"=u32 250) -> ("Timeout"=w336:bool)  [unwired: 8 in, 1 out]
                  n175 = call-poly <vilib>:"WPI_RobotDriveArcadeDrive.vi"("Y axis value"=-0.6, "X axis value"=0.0, "RobotDriveDevRef"=w333) -> ("RobotDriveDevRef"=w332:T6)  [unwired: 6 in, 2 out]
                }
                n176 = while {
                  tunnel: w292 -> [w345]
                  tunnel: [w345] -> w293
                  tunnel: w299 -> [w343]
                  tunnel: w295 -> [w342]
                  tunnel: w294 -> [w339]
                  stop <- w346 stop-if-true
                  n177 = call <vilib>:"WPI_PotentiometerGetNormalized.vi"("PotDevRef"=w342) -> ("Normalized Value"=w341:dbl)  [unwired: 8 in, 2 out]
                  n178 = disable-structure shown="Enabled" {
                    disable-tunnel: w341 -> [w349 w352]
                    disable-tunnel: [w348 w350] -> w340
                    disable-tunnel: w339 -> [_ w351]
                    frame Disabled {
                      n179 = expression code="-1505.88*(x-.587)"(w349) -> (w348:dbl)
                    }
                    frame Enabled {
                      n180 = Subtract(x=w352, y=w351) -> (x-y=w354:dbl)
                      n181 = Multiply(x=w354, y=-1505.88) -> (x*y=w350:dbl)
                    }
                  }
                  n182 = Less Or Equal?(x=w340, y=300.0) -> (x <= y?=w346:bool)
                  n183 = call-poly <vilib>:"WPI_RobotDriveArcadeDrive.vi"("Y axis value"=-0.45, "RobotDriveDevRef"=w343) -> ()  [unwired: 7 in, 3 out]
                }
                n184 = call "Set Arm Position.vi"("RobotDriveDevRef 2"=w292, "Speed"=0.8, "Setpoint"=150.0) -> ()  [unwired: 8 in, 1 out]
                n185 = disable-structure shown="Enabled" {
                  disable-tunnel: [w312 w324] -> w298
                  disable-tunnel: w293 -> [w311 w325]
                  frame Disabled {
                    # "Go forward"
                    n186 = Tick Count (ms)() -> (millisecond timer value=w316:u32)
                    n187 = while {
                      tunnel: w316 -> [w323]
                      tunnel: [24.0 ("Distance")] -> w313
                      stop <- w321 stop-if-true
                      n188 = call "Timeout.vi"("Start Time In"=w323, "Time Limit"=u32 10000) -> ("Timeout"=w321:bool)  [unwired: 8 in, 1 out]
                    }
                    n189 = call "Forward For inch.vi"("Angle"=0.0 ("Angle robot facing"), "Speed"=-0.7, "Distance"=60.0, "drive.lvclass"=w311) -> ("drive.lvclass"=w312:refnum<class "drive.lvclass">)  [unwired: 7 in]
                    n190 = call "Forward For inch.vi"("Angle"=0.0 ("Angle robot facing"), "Speed"=-0.65, "Distance"=w313, "drive.lvclass"=w312) -> ()  [unwired: 7 in, 1 out]
                  }
                  frame Enabled {
                    n191 = for {
                      N: 150 -> [_]
                      tunnel: w325 -> [w329]
                      tunnel: [w327] -> w324
                      n192 = call-poly <vilib>:"WPI_RobotDriveArcadeDrive.vi"("Y axis value"=-0.7, "X axis value"=0.0, "RobotDriveDevRef"=w329) -> ("RobotDriveDevRef"=w327:T6)  [unwired: 6 in, 2 out]
                      n193 = Wait (ms)(milliseconds to wait=u32 20) -> ()  [unwired: 1 out]
                    }
                  }
                }
              }
              frame Enabled {
                # "Go forward"
                # "Wait"
                # "Raise arm"
                # "Forward"
                # "Pause"
                # "Forward"
                # "Lower arm"
                # "Pause"
                n194 = for {
                  N: 1 -> [_]
                  tunnel: w375 -> [w402]
                  tunnel: [w402] -> w371
                  n195 = Wait (ms)(milliseconds to wait=u32 750) -> ()  [unwired: 1 out]
                }
                n196 = call <vilib>:"WPI_SwitchRefNum Registry Get.vi"("refnum name"="mechanismSwitch") -> ("SwitchDevRef"=w379:T14)  [unwired: 9 in, 1 out]
                n197 = call <vilib>:"WPI_RobotDriveRefNum Registry Get.vi"("refnum name"="intakeDevice") -> ("RobotDriveDevRef"=w378:T6)  [unwired: 9 in, 1 out]
                n198 = for {
                  N: 60 -> [_]
                  tunnel: w379 -> [w407]
                  tunnel: w378 -> [w406]
                  tunnel: w375 -> [_]
                  stop <- w405 stop-if-true
                  n199 = call <vilib>:"WPI_SwitchGetLimitValue.vi"("SwitchDevRef"=w407) -> ("Switch Pressed"=w405:bool)  [unwired: 8 in, 2 out]
                  n200 = call-poly <vilib>:"WPI_RobotDriveArcadeDrive.vi"("Y axis value"=-0.7, "X axis value"=0.0, "RobotDriveDevRef"=w406) -> ()  [unwired: 6 in, 3 out]
                  n201 = Wait (ms)(milliseconds to wait=u32 50) -> ()  [unwired: 1 out]
                }
                n202 = call "Forward For inch.vi"("Angle"=0.0 ("Angle robot facing"), "Speed"=-0.6, "Distance"=46.0, "drive.lvclass"=w371) -> ("drive.lvclass"=w369:refnum<class "drive.lvclass">)  [unwired: 7 in]
                n203 = for {
                  N: 1 -> [_]
                  tunnel: w369 -> [w400]
                  tunnel: [w400] -> w368
                  n204 = Wait (ms)(milliseconds to wait=u32 200) -> ()  [unwired: 1 out]
                }
                n205 = for {
                  N: 6 -> [_]
                  tunnel: w368 -> [w384]
                  tunnel: [w383] -> w363
                  n206 = Wait (ms)(milliseconds to wait=u32 50) -> ()  [unwired: 1 out]
                  n207 = call-poly <vilib>:"WPI_RobotDriveArcadeDrive.vi"("Y axis value"=-0.6, "X axis value"=0.0, "RobotDriveDevRef"=w384) -> ("RobotDriveDevRef"=w383:T6)  [unwired: 6 in, 2 out]
                }
                n208 = call <vilib>:"WPI_RobotDriveRefNum Registry Get.vi"("refnum name"="intakeDevice") -> ("RobotDriveDevRef"=w365:T6)  [unwired: 9 in, 1 out]
                n209 = for {
                  N: 50 -> [_]
                  tunnel: w363 -> [_]
                  tunnel: w365 -> [w396]
                  n210 = call-poly <vilib>:"WPI_RobotDriveArcadeDrive.vi"("Y axis value"=0.8, "X axis value"=0.0, "RobotDriveDevRef"=w396) -> ()  [unwired: 6 in, 3 out]
                  n211 = Wait (ms)(milliseconds to wait=u32 50) -> ()  [unwired: 1 out]
                }
                n212 = for {
                  N: 40 -> [_]
                  tunnel: w363 -> [w392]
                  tunnel: [w392] -> w361
                  n213 = Wait (ms)(milliseconds to wait=u32 20) -> ()  [unwired: 1 out]
                  n214 = call-poly <vilib>:"WPI_RobotDriveArcadeDrive.vi"("Y axis value"=-0.55, "X axis value"=0.0, "RobotDriveDevRef"=w392) -> ()  [unwired: 6 in, 3 out]
                }
                n215 = for {
                  N: 90 -> [_]
                  tunnel: w361 -> [w389]
                  tunnel: [w387] -> w360
                  n216 = call-poly <vilib>:"WPI_RobotDriveArcadeDrive.vi"("Y axis value"=-0.85, "X axis value"=0.0, "RobotDriveDevRef"=w389) -> ("RobotDriveDevRef"=w387:T6)  [unwired: 6 in, 2 out]
                  n217 = Wait (ms)(milliseconds to wait=u32 20) -> ()  [unwired: 1 out]
                }
              }
            }
          }
          frame 3 {
            # "CDF"
            n218 = disable-structure shown="Enabled" {
              disable-tunnel: w411 -> [w426 w456]
              disable-tunnel: [w412 w442] -> w410
              frame Disabled {
                # "Raise arm so it doesn't hit the ground"
                # "Go over"
                # "Very small pause"
                # "While going forward so\nwe don't roll off"
                # "Lower arm onto CDF"
                # "Forward"
                n219 = call "Forward For inch.vi"("Angle"=0.0 ("Angle robot facing"), "Speed"=-0.6, "Distance"=38.5, "drive.lvclass"=w426) -> ("drive.lvclass"=w417:refnum<class "drive.lvclass">)  [unwired: 7 in]
                n220 = call "Set Arm Position.vi"("RobotDriveDevRef 2"=w417, "Speed"=0.9, "Setpoint"=650.0) -> ("RobotDriveDevRef"=w416:T6)  [unwired: 8 in]
                n221 = for {
                  N: 50 -> [_]
                  tunnel: w417 -> [w429]
                  n222 = Wait (ms)(milliseconds to wait=u32 20) -> ()  [unwired: 1 out]
                  n223 = call-poly <vilib>:"WPI_RobotDriveArcadeDrive.vi"("Y axis value"=-0.35, "X axis value"=0.0 ("Y axis value"), "RobotDriveDevRef"=w429) -> ()  [unwired: 6 in, 3 out]
                }
                n224 = Tick Count (ms)() -> (millisecond timer value=w413:u32)
                n225 = for {
                  N: 5 -> [_]
                  tunnel: [w427] -> w418
                  tunnel: w416 -> [w427]
                  n226 = Wait (ms)(milliseconds to wait=u32 50) -> ()  [unwired: 1 out]
                }
                n227 = while {
                  tunnel: w416 -> [w440]
                  tunnel: [w439] -> w412
                  tunnel: w413 -> [w436]
                  stop <- w435 stop-if-true
                  n228 = call "Timeout.vi"("Start Time In"=w436, "Time Limit"=u32 4000) -> ("Timeout"=w435:bool)  [unwired: 8 in, 1 out]
                  n229 = call "Drive Straight.vi"("Angle robot facing"=0.0) -> ("Arcade drive x"=w433:dbl)  [unwired: 9 in, 1 out]
                  n230 = call-poly <vilib>:"WPI_RobotDriveArcadeDrive.vi"("Y axis value"=-0.65, "X axis value"=w433, "RobotDriveDevRef"=w440) -> ("RobotDriveDevRef"=w439:T6)  [unwired: 6 in, 2 out]
                  n231 = Wait (ms)(milliseconds to wait=u32 20) -> ()  [unwired: 1 out]
                }
                n232 = call "Set Arm Position.vi"("RobotDriveDevRef 2"=w418, "Speed"=0.9, "Setpoint"=200.0) -> ()  [unwired: 8 in, 1 out]
              }
              frame Enabled {
                # "forward"
                # "arm up"
                # "While going forward so\nwe don't roll off"
                n233 = call "Forward For inch.vi"("Angle"=0.0 ("Angle robot facing"), "Speed"=-0.6, "Distance"=38.0, "drive.lvclass"=w456) -> ("drive.lvclass"=w452:refnum<class "drive.lvclass">)  [unwired: 7 in]
                n234 = call <vilib>:"WPI_SwitchRefNum Registry Get.vi"("refnum name"="mechanismSwitch") -> ("SwitchDevRef"=w449:T14)  [unwired: 9 in, 1 out]
                n235 = for {
                  N: 50 -> [_]
                  tunnel: w452 -> [w484]
                  n236 = Wait (ms)(milliseconds to wait=u32 20) -> ()  [unwired: 1 out]
                  n237 = call-poly <vilib>:"WPI_RobotDriveArcadeDrive.vi"("Y axis value"=-0.35, "X axis value"=0.0 ("Y axis value"), "RobotDriveDevRef"=w484) -> ()  [unwired: 6 in, 3 out]
                }
                n238 = call <vilib>:"WPI_RobotDriveRefNum Registry Get.vi"("refnum name"="intakeDevice") -> ("RobotDriveDevRef"=w453:T6)  [unwired: 9 in, 1 out]
                n239 = for {
                  N: 50 -> [_]
                  tunnel: w453 -> [w480]
                  tunnel: w452 -> [w476]
                  tunnel: w449 -> [w478]
                  tunnel: [w477] -> w447
                  tunnel: [w476] -> w443
                  stop <- w479 stop-if-true
                  n240 = call <vilib>:"WPI_SwitchGetLimitValue.vi"("SwitchDevRef"=w478) -> ("Switch Pressed"=w479:bool)  [unwired: 8 in, 2 out]
                  n241 = call-poly <vilib>:"WPI_RobotDriveArcadeDrive.vi"("Y axis value"=-0.8, "X axis value"=0.0, "RobotDriveDevRef"=w480) -> ("RobotDriveDevRef"=w477:T6)  [unwired: 6 in, 2 out]
                  n242 = Wait (ms)(milliseconds to wait=u32 50) -> ()  [unwired: 1 out]
                }
                n243 = Tick Count (ms)() -> (millisecond timer value=w444:u32)
                n244 = while {
                  tunnel: w443 -> [w460]
                  tunnel: [w467] -> w442
                  tunnel: w444 -> [w464]
                  stop <- w463 stop-if-true
                  n245 = call "Timeout.vi"("Start Time In"=w464, "Time Limit"=u32 5000) -> ("Timeout"=w463:bool)  [unwired: 8 in, 1 out]
                  n246 = call "Drive Straight.vi"("Angle robot facing"=0.0, "drive.lvclass"=w460) -> ("Arcade drive x"=w461:dbl)  [unwired: 8 in, 1 out]
                  n247 = call-poly <vilib>:"WPI_RobotDriveArcadeDrive.vi"("Y axis value"=-0.7, "X axis value"=w461, "RobotDriveDevRef"=w460) -> ("RobotDriveDevRef"=w467:T6)  [unwired: 6 in, 2 out]
                  n248 = Wait (ms)(milliseconds to wait=u32 40) -> ()  [unwired: 1 out]
                }
                n249 = for {
                  N: 5 -> [_]
                  tunnel: [w474] -> w446
                  tunnel: w447 -> [w474]
                  n250 = Wait (ms)(milliseconds to wait=u32 50) -> ()  [unwired: 1 out]
                }
                n251 = for {
                  N: 25 -> [_]
                  tunnel: w446 -> [w470]
                  tunnel: [w469] -> _
                  n252 = call-poly <vilib>:"WPI_RobotDriveArcadeDrive.vi"("Y axis value"=0.7, "X axis value"=0.0, "RobotDriveDevRef"=w470) -> ("RobotDriveDevRef"=w469:T6)  [unwired: 6 in, 2 out]
                  n253 = Wait (ms)(milliseconds to wait=u32 50) -> ()  [unwired: 1 out]
                }
              }
            }
          }
          frame 4 {
            # "Turn to the left, so right wheel hits\nedge of rampart. It is easier to go over\nthis way"
            # "Go forward"
            # "RAMPARTS"
            n254 = disable-structure shown="Disabled" {
              disable-tunnel: w494 -> [w499 _]
              frame Disabled {
                # "Raise arm a little"
                n255 = call "Set Arm Position.vi"("RobotDriveDevRef 2"=w499, "Setpoint"=100.0) -> ()  [unwired: 9 in, 1 out]
              }
              frame Enabled {
              }
            }
            n256 = call "Forward For inch.vi"("Angle"=0.0 ("Angle robot facing"), "Speed"=-0.65, "Distance"=30.0, "drive.lvclass"=w494) -> ("drive.lvclass"=w488:refnum<class "drive.lvclass">)  [unwired: 7 in]
            n257 = call "Turn To Angle.vi"("Speed/Direction"=0.63, "Angle"=-7.0, "drive.lvclass"=w488) -> ("drive.lvclass"=w497:refnum<class "drive.lvclass">, 7:w493)  [unwired: 7 in]
            n258 = Tick Count (ms)() -> (millisecond timer value=w489:u32)
            n259 = while {
              tunnel: [w508] -> w498
              tunnel: w497 -> [w504]
              tunnel: w489 -> [w502]
              stop <- w501 stop-if-true
              # "Forward until over"
              n260 = call "Timeout.vi"("Start Time In"=w502, "Time Limit"=u32 4000) -> ("Timeout"=w501:bool)  [unwired: 8 in, 1 out]
              n261 = call "Drive Straight.vi"("Angle robot facing"=-5.0) -> ("Arcade drive x"=w506:dbl)  [unwired: 9 in, 1 out]
              n262 = Wait (ms)(milliseconds to wait=u32 20) -> ()  [unwired: 1 out]
              n263 = call-poly <vilib>:"WPI_RobotDriveArcadeDrive.vi"("Y axis value"=-0.68, "X axis value"=w506, "RobotDriveDevRef"=w504) -> ("RobotDriveDevRef"=w508:T6)  [unwired: 6 in, 2 out]
            }
          }
          frame 5 {
            # "MOAT"
            n264 = Tick Count (ms)() -> (millisecond timer value=w510:u32)
            n265 = disable-structure shown="Disabled" {
              disable-tunnel: w511 -> [w513 _]
              frame Disabled {
                # "Raise arm"
                n266 = call "Set Arm Position.vi"("RobotDriveDevRef 2"=w513, "Setpoint"=50.0) -> ()  [unwired: 9 in, 1 out]
              }
              frame Enabled {
              }
            }
            n267 = while {
              tunnel: w511 -> [w521]
              tunnel: [w522] -> w512
              tunnel: w510 -> [w517]
              stop <- w515 stop-if-true
              # "Go forward"
              n268 = call "Timeout.vi"("Start Time In"=w517, "Time Limit"=u32 5000) -> ("Timeout"=w515:bool)  [unwired: 8 in, 1 out]
              n269 = call "Drive Straight.vi"("Angle robot facing"=0.0) -> ("Arcade drive x"=w518:dbl)  [unwired: 9 in, 1 out]
              n270 = call-poly <vilib>:"WPI_RobotDriveArcadeDrive.vi"("Y axis value"=-0.75, "X axis value"=w518, "RobotDriveDevRef"=w521) -> ("RobotDriveDevRef"=w522:T6)  [unwired: 6 in, 2 out]
              n271 = Wait (ms)(milliseconds to wait=u32 20) -> ()  [unwired: 1 out]
            }
          }
          frame 6 {
            # "DRAWBRIDGE"
            n272 = Tick Count (ms)() -> (millisecond timer value=w524:u32)
            n273 = while {
              tunnel: w525 -> [w531]
              tunnel: [w532] -> w526
              tunnel: w524 -> [w528]
              stop <- w527 stop-if-true
              n274 = call "Timeout.vi"("Start Time In"=w528, "Time Limit"=u32 4000) -> ("Timeout"=w527:bool)  [unwired: 8 in, 1 out]
              n275 = call-poly <vilib>:"WPI_RobotDriveArcadeDrive.vi"("Y axis value"=-0.6, "X axis value"=0.0 ("Y axis value"), "RobotDriveDevRef"=w531) -> ("RobotDriveDevRef"=w532:T6)  [unwired: 6 in, 2 out]
              n276 = Wait (ms)(milliseconds to wait=u32 20) -> ()  [unwired: 1 out]
            }
          }
          frame 7 {
            # "SALLY PORT"
            n277 = Tick Count (ms)() -> (millisecond timer value=w537:u32)
            n278 = while {
              tunnel: w536 -> [w542]
              tunnel: [w543] -> w535
              tunnel: w537 -> [w539]
              stop <- w538 stop-if-true
              n279 = call "Timeout.vi"("Start Time In"=w539, "Time Limit"=u32 4000) -> ("Timeout"=w538:bool)  [unwired: 8 in, 1 out]
              n280 = call-poly <vilib>:"WPI_RobotDriveArcadeDrive.vi"("Y axis value"=-0.6, "X axis value"=0.0 ("Y axis value"), "RobotDriveDevRef"=w542) -> ("RobotDriveDevRef"=w543:T6)  [unwired: 6 in, 2 out]
              n281 = Wait (ms)(milliseconds to wait=u32 20) -> ()  [unwired: 1 out]
            }
          }
          frame 8 {
            # "ROCK WALL"
            # "Forward fast\nto save time"
            n282 = call "Forward For inch.vi"("Angle"=0.0 ("Angle robot facing"), "Speed"=-0.85, "Distance"=35.0, "drive.lvclass"=w551) -> ("drive.lvclass"=w550:refnum<class "drive.lvclass">)  [unwired: 7 in]
            n283 = disable-structure shown="Disabled" {
              disable-tunnel: w551 -> [w553 _]
              frame Disabled {
                n284 = call "Set Arm Position.vi"("RobotDriveDevRef 2"=w553, "Setpoint"=50.0) -> ()  [unwired: 9 in, 1 out]
              }
              frame Enabled {
              }
            }
            n285 = Tick Count (ms)() -> (millisecond timer value=w546:u32)
            n286 = while {
              tunnel: w550 -> [w561]
              tunnel: [w562] -> w552
              tunnel: w546 -> [w555]
              stop <- w556 stop-if-true
              # "Forward"
              n287 = call "Timeout.vi"("Start Time In"=w555, "Time Limit"=u32 3500) -> ("Timeout"=w556:bool)  [unwired: 8 in, 1 out]
              n288 = call "Drive Straight.vi"("Angle robot facing"=0.0) -> ("Arcade drive x"=w559:dbl)  [unwired: 9 in, 1 out]
              n289 = call-poly <vilib>:"WPI_RobotDriveArcadeDrive.vi"("Y axis value"=-0.65, "X axis value"=w559, "RobotDriveDevRef"=w561) -> ("RobotDriveDevRef"=w562:T6)  [unwired: 6 in, 2 out]
              n290 = Wait (ms)(milliseconds to wait=u32 20) -> ()  [unwired: 1 out]
            }
          }
          frame 9 {
            n291 = Tick Count (ms)() -> (millisecond timer value=w565:u32)
            n292 = disable-structure shown="Disabled" {
              disable-tunnel: w566 -> [w567 _]
              frame Disabled {
                # "Arm up"
                # "ROUGH TERRAIN"
                n293 = call "Set Arm Position.vi"("RobotDriveDevRef 2"=w567, "Setpoint"=100.0) -> ()  [unwired: 9 in, 1 out]
              }
              frame Enabled {
              }
            }
            n294 = while {
              tunnel: w566 -> [w575]
              tunnel: [w576] -> w564
              tunnel: w565 -> [w570]
              stop <- w569 stop-if-true
              # "Go forward"
              n295 = call "Timeout.vi"("Start Time In"=w570, "Time Limit"=u32 4000) -> ("Timeout"=w569:bool)  [unwired: 8 in, 1 out]
              n296 = call "Drive Straight.vi"("Angle robot facing"=0.0) -> ("Arcade drive x"=w573:dbl)  [unwired: 9 in, 1 out]
              n297 = Wait (ms)(milliseconds to wait=u32 20) -> ()  [unwired: 1 out]
              n298 = call-poly <vilib>:"WPI_RobotDriveArcadeDrive.vi"("Y axis value"=-0.65, "X axis value"=w573, "RobotDriveDevRef"=w575) -> ("RobotDriveDevRef"=w576:T6)  [unwired: 6 in, 2 out]
            }
          }
        }
        n299 = flat-sequence {
          tunnel: w233 -> [_]
          frame #0 {
            n300 = local write "Stop Wheel Loop"(TRUE) -> ()
          }
        }
        n301 = call-poly <vilib>:"NT Read Value.vi"("Name"="Shoot") -> ("Boolean"=w225:bool)  [unwired: 9 in, 1 out]
        n302 = call-poly <vilib>:"NT Read Value.vi"("Name"="Defense Position") -> ("Numeric"=w224:dbl)  [unwired: 9 in, 1 out]
        n303 = case shown="True" w225 {
          tunnel: w224 -> [_ w666]
          tunnel: w221 -> [w578 w665]
          tunnel: w227 -> [_ w663]
          tunnel: w223 -> [_ w662]
          frame False {
            n304 = call-poly <vilib>:"NT Read Value.vi"("Name"="Cross Back") -> ("Boolean"=w580:bool)  [unwired: 9 in, 1 out]
            n305 = case shown="False" w580 {
              tunnel: w578 -> [_ w585]
              frame False {
                n306 = call-poly <vilib>:"NT Write Value.vi"("Numeric"=3.0, "Name"="Template") -> ()  [unwired: 9 in, 1 out]
              }
              frame True {
                n307 = Tick Count (ms)() -> (millisecond timer value=w584:u32)
                n308 = while {
                  tunnel: w584 -> [w591]
                  tunnel: [w588] -> w583
                  stop <- w590 stop-if-true
                  w588 = u32 20 ("milliseconds to wait")
                  n309 = Wait (ms)(milliseconds to wait=w588) -> ()  [unwired: 1 out]
                  n310 = call "Timeout.vi"("Start Time In"=w591, "Time Limit"=u32 500 ("milliseconds to wait")) -> ("Timeout"=w590:bool)  [unwired: 8 in, 1 out]
                }
                n311 = call-poly <vilib>:"NT Read Value.vi"("Name"="Defense") -> ("Numeric"=w586:dbl)  [unwired: 9 in, 1 out]
                n312 = case shown="1" w586 {
                  tunnel: w585 -> [_ w593 _ _ w599 w609 w620 w630 w640 w651]
                  tunnel: w583 -> [_ _ _ _ _ _ _ _ _ _]
                  frame 0, Default {
                  }
                  frame 1 {
                    # "LOW BAR"
                    # "in front of outer works\nto neutral zone"
                    # "drive forward from castle \nwall to outer works"
                    n313 = call "Set Arm Position.vi"("RobotDriveDevRef 2"=w593, "Speed"=0.8, "Setpoint"=600.0) -> ("RobotDriveDevRef"=w592:T6)  [unwired: 8 in]
                    n314 = call "Forward For inch.vi"("Angle"=0.0 ("Angle robot facing"), "Speed"=-0.65, "Distance"=192.0, "drive.lvclass"=w592) -> ()  [unwired: 7 in, 1 out]
                  }
                  frame 2 {
                    # "PORTCULLIS"
                    # "NOT WORTH IT"
                    # "NO"
                  }
                  frame 3 {
                    # "CDF"
                    # "NOT WORTH IT EITHER, CROSSING IS GOOD ENOUGH"
                  }
                  frame 4 {
                    # "RAMPARTS"
                    n315 = Tick Count (ms)() -> (millisecond timer value=w600:u32)
                    n316 = while {
                      tunnel: w600 -> [w603]
                      tunnel: w599 -> [w601]
                      stop <- w602 stop-if-true
                      # "Forward until over"
                      n317 = call "Timeout.vi"("Start Time In"=w603, "Time Limit"=u32 3000) -> ("Timeout"=w602:bool)  [unwired: 8 in, 1 out]
                      n318 = call "Drive Straight.vi"("Angle robot facing"=-5.0) -> ("Arcade drive x"=w606:dbl)  [unwired: 9 in, 1 out]
                      n319 = Wait (ms)(milliseconds to wait=u32 20) -> ()  [unwired: 1 out]
                      n320 = call-poly <vilib>:"WPI_RobotDriveArcadeDrive.vi"("Y axis value"=0.68, "X axis value"=w606, "RobotDriveDevRef"=w601) -> ()  [unwired: 6 in, 3 out]
                    }
                  }
                  frame 5 {
                    # "MOAT"
                    n321 = Tick Count (ms)() -> (millisecond timer value=w610:u32)
                    n322 = while {
                      tunnel: w609 -> [w617]
                      tunnel: [w618] -> _
                      tunnel: w610 -> [w613]
                      stop <- w611 stop-if-true
                      # "Go forward"
                      n323 = call "Timeout.vi"("Start Time In"=w613, "Time Limit"=u32 4000) -> ("Timeout"=w611:bool)  [unwired: 8 in, 1 out]
                      n324 = call "Drive Straight.vi"("Angle robot facing"=0.0) -> ("Arcade drive x"=w614:dbl)  [unwired: 9 in, 1 out]
                      n325 = call-poly <vilib>:"WPI_RobotDriveArcadeDrive.vi"("Y axis value"=0.75, "X axis value"=w614, "RobotDriveDevRef"=w617) -> ("RobotDriveDevRef"=w618:T6)  [unwired: 6 in, 2 out]
                      n326 = Wait (ms)(milliseconds to wait=u32 20) -> ()  [unwired: 1 out]
                    }
                  }
                  frame 6 {
                    # "DRAWBRIDGE"
                    n327 = Tick Count (ms)() -> (millisecond timer value=w621:u32)
                    n328 = while {
                      tunnel: w620 -> [w626]
                      tunnel: [w627] -> _
                      tunnel: w621 -> [w623]
                      stop <- w622 stop-if-true
                      n329 = call "Timeout.vi"("Start Time In"=w623, "Time Limit"=u32 3000) -> ("Timeout"=w622:bool)  [unwired: 8 in, 1 out]
                      n330 = call-poly <vilib>:"WPI_RobotDriveArcadeDrive.vi"("Y axis value"=0.6, "X axis value"=0.0 ("Y axis value"), "RobotDriveDevRef"=w626) -> ("RobotDriveDevRef"=w627:T6)  [unwired: 6 in, 2 out]
                      n331 = Wait (ms)(milliseconds to wait=u32 20) -> ()  [unwired: 1 out]
                    }
                  }
                  frame 7 {
                    # "SALLY PORT"
                    n332 = Tick Count (ms)() -> (millisecond timer value=w631:u32)
                    n333 = while {
                      tunnel: w630 -> [w636]
                      tunnel: [w637] -> _
                      tunnel: w631 -> [w633]
                      stop <- w632 stop-if-true
                      n334 = call "Timeout.vi"("Start Time In"=w633, "Time Limit"=u32 3000) -> ("Timeout"=w632:bool)  [unwired: 8 in, 1 out]
                      n335 = call-poly <vilib>:"WPI_RobotDriveArcadeDrive.vi"("Y axis value"=0.6, "X axis value"=0.0 ("Y axis value"), "RobotDriveDevRef"=w636) -> ("RobotDriveDevRef"=w637:T6)  [unwired: 6 in, 2 out]
                      n336 = Wait (ms)(milliseconds to wait=u32 20) -> ()  [unwired: 1 out]
                    }
                  }
                  frame 8 {
                    # "ROCK WALL"
                    n337 = Tick Count (ms)() -> (millisecond timer value=w641:u32)
                    n338 = while {
                      tunnel: w640 -> [w648]
                      tunnel: [w649] -> _
                      tunnel: w641 -> [w642]
                      stop <- w643 stop-if-true
                      # "Forward"
                      n339 = call "Timeout.vi"("Start Time In"=w642, "Time Limit"=u32 2500) -> ("Timeout"=w643:bool)  [unwired: 8 in, 1 out]
                      n340 = call "Drive Straight.vi"("Angle robot facing"=0.0) -> ("Arcade drive x"=w646:dbl)  [unwired: 9 in, 1 out]
                      n341 = call-poly <vilib>:"WPI_RobotDriveArcadeDrive.vi"("Y axis value"=0.65, "X axis value"=w646, "RobotDriveDevRef"=w648) -> ("RobotDriveDevRef"=w649:T6)  [unwired: 6 in, 2 out]
                      n342 = Wait (ms)(milliseconds to wait=u32 20) -> ()  [unwired: 1 out]
                    }
                  }
                  frame 9 {
                    n343 = Tick Count (ms)() -> (millisecond timer value=w652:u32)
                    n344 = while {
                      tunnel: [w660] -> _
                      tunnel: w652 -> [w655]
                      tunnel: w651 -> [w653]
                      stop <- w654 stop-if-true
                      # "Go forward"
                      n345 = call "Timeout.vi"("Start Time In"=w655, "Time Limit"=u32 4000) -> ("Timeout"=w654:bool)  [unwired: 8 in, 1 out]
                      n346 = call "Drive Straight.vi"("Angle robot facing"=0.0) -> ("Arcade drive x"=w658:dbl)  [unwired: 9 in, 1 out]
                      n347 = Wait (ms)(milliseconds to wait=u32 20) -> ()  [unwired: 1 out]
                      n348 = call-poly <vilib>:"WPI_RobotDriveArcadeDrive.vi"("Y axis value"=0.65, "X axis value"=w658, "RobotDriveDevRef"=w653) -> ("RobotDriveDevRef"=w660:T6)  [unwired: 6 in, 2 out]
                    }
                  }
                }
              }
            }
          }
          frame True {
            n349 = case shown="3" w666 {
              tunnel: w665 -> [_ w690 w786 w887 w975 w989]
              tunnel: w662 -> [_ w681 w777 w897 _ w990]
              frame 0, Default {
              }
              frame 1 {
                # "disabled case for driving to wall\n at an angle"
                # "disabled case for driving to wall\nat an angle"
                # "Raise arm so it doesn't\ndrag on ground"
                # "This ensures that the intake wheels spit out the boulder with\none second left in auto, no matter if the other\nactions (the last turning part is our real concern) finish."
                # "Lower arm"
                # "Shoot"
                n350 = disable-structure shown="Disabled" {
                  disable-tunnel: w690 -> [w736 _]
                  frame Disabled {
                    n351 = call "Set Arm Position.vi"("RobotDriveDevRef 2"=w736, "Speed"=0.8, "Setpoint"=480.0) -> ()  [unwired: 8 in, 1 out]
                  }
                  frame Enabled {
                  }
                }
                n352 = call <vilib>:"WPI_AccelerometerRefNum Registry Get.vi"("refnum name"="accel") -> ("AccelerometerDevRef"=w695:T17)  [unwired: 9 in, 1 out]
                n353 = while {
                  tunnel: w681 -> [w710]
                  tunnel: [w709] -> w680
                  stop <- w709 stop-if-true
                  n354 = call "Timeout.vi"("Start Time In"=w710, "Time Limit"=u32 14000) -> ("Timeout"=w709:bool)  [unwired: 8 in, 1 out]
                  n355 = Wait (ms)(milliseconds to wait=u32 300) -> ()  [unwired: 1 out]
                }
                n356 = Tick Count (ms)() -> (millisecond timer value=w687:u32)
                n357 = while {
                  tunnel: w695 -> [w756]
                  tunnel: w690 -> [w748]
                  tunnel: [w747] -> w684
                  tunnel: [w746] -> _
                  tunnel: w687 -> [w743]
                  stop <- w745 stop-if-true
                  n358 = disable-structure shown="Enabled" {
                    disable-tunnel: [w759 0.0 ("X axis value")] -> w741
                    disable-tunnel: [u32 10000 ("Time Limit") u32 10000 ("Time Limit")] -> w740
                    frame Enabled {
                      n359 = call "Drive Straight.vi"("Angle robot facing"=10.0) -> ("Arcade drive x"=w759:dbl)  [unwired: 9 in, 1 out]
                    }
                    frame Disabled {
                    }
                  }
                  n360 = call <vilib>:"WPI_AccelerometerGetAcceleration.vi"("AccelerometerDevRef"=w756) -> ("Accelerations"=w755:T23, "AccelerometerDevRef"=w746:T17)  [unwired: 8 in, 1 out]
                  n361 = call "Timeout.vi"("Start Time In"=w743, "Time Limit"=w740) -> ("Timeout"=w742:bool)  [unwired: 8 in, 1 out]
                  n362 = Unbundle By Name(w755) -> ("Y-Axis"=w751:dbl)
                  n363 = In Range and Coerce(upper limit=0.8, x=w751, lower limit=-0.8) -> (In Range?=w752:bool)  [unwired: 1 out]
                  n364 = Not(x=w752) -> (.not. x?=w744:bool)
                  n365 = call-poly <vilib>:"WPI_RobotDriveArcadeDrive.vi"("Y axis value"=0.65, "X axis value"=w741, "RobotDriveDevRef"=w748) -> ("RobotDriveDevRef"=w747:T6)  [unwired: 6 in, 2 out]
                  n366 = Or(x=w744, y=w742) -> (x .or. y?=w745:bool)
                  n367 = Wait (ms)(milliseconds to wait=u32 20) -> ()  [unwired: 1 out]
                }
                n368 = disable-structure shown="Disabled" {
                  frame Disabled {
                    n369 = call "Turn And Shoot.vi"("Turning Angle"=-95.0) -> ()  [unwired: 11 in]
                  }
                  frame Enabled {
                  }
                }
                n370 = for {
                  N: 1 -> [_]
                  tunnel: [w729] -> w683
                  tunnel: w684 -> [w729]
                  n371 = Wait (ms)(milliseconds to wait=u32 350) -> ()  [unwired: 1 out]
                }
                n372 = call <vilib>:"WPI_RobotDriveRefNum Registry Get.vi"("refnum name"="intakeDevice") -> ("RobotDriveDevRef"=w672:T6)  [unwired: 9 in, 1 out]
                n373 = call "Forward For inch.vi"("Angle"=0.0 ("Angle robot facing"), "Speed"=-0.6, "Distance"=2.0, "drive.lvclass"=w683) -> ("drive.lvclass"=w670:refnum<class "drive.lvclass">)  [unwired: 7 in]
                n374 = for {
                  N: 40 -> [_]
                  tunnel: w672 -> [w703]
                  tunnel: w670 -> [_]
                  tunnel: [w701] -> w667
                  n375 = call-poly <vilib>:"WPI_RobotDriveArcadeDrive.vi"("Y axis value"=0.6, "X axis value"=0.0, "RobotDriveDevRef"=w703) -> ("RobotDriveDevRef"=w701:T6)  [unwired: 6 in, 2 out]
                  n376 = Wait (ms)(milliseconds to wait=u32 20) -> ()  [unwired: 1 out]
                }
                n377 = disable-structure shown="Enabled" {
                  disable-tunnel: [-100.0 ("Angle") -90.0 ("Angle")] -> w675
                  frame Disabled {
                  }
                  frame Enabled {
                  }
                }
                n378 = call "Turn To Angle.vi"(7:w670, "Speed/Direction"=-0.9, "Angle"=w675) -> ("drive.lvclass"=w668:refnum<class "drive.lvclass">)  [unwired: 8 in]
                n379 = call-poly <vilib>:"NT Write Value.vi"("Numeric"=3.0, "Name"="Template") -> ()  [unwired: 9 in, 1 out]
                n380 = for {
                  N: 30 -> [_]
                  tunnel: w667 -> [w698]
                  tunnel: w668 -> [_]
                  n381 = call-poly <vilib>:"WPI_RobotDriveArcadeDrive.vi"("Y axis value"=-0.5, "X axis value"=0.0, "RobotDriveDevRef"=w698) -> ()  [unwired: 6 in, 3 out]
                  n382 = Wait (ms)(milliseconds to wait=u32 20) -> ()  [unwired: 1 out]
                }
                n383 = disable-structure shown="Enabled" {
                  disable-tunnel: w668 -> [w713 w718]
                  disable-tunnel: [w712 w717] -> w682
                  frame Disabled {
                    n384 = call "Forward For inch.vi"("Angle"=-90.0 ("Angle robot facing"), "Speed"=-0.6, "Distance"=72.0, "drive.lvclass"=w713) -> ("drive.lvclass"=w712:refnum<class "drive.lvclass">)  [unwired: 7 in]
                  }
                  frame Enabled {
                    n385 = disable-structure shown="Disabled" {
                      disable-tunnel: w718 -> [w722 _]
                      frame Disabled {
                        n386 = call "Set Arm Position.vi"("RobotDriveDevRef 2"=w722, "Speed"=0.8, "Setpoint"=550.0) -> ()  [unwired: 8 in, 1 out]
                      }
                      frame Enabled {
                      }
                    }
                    n387 = for {
                      N: 50 -> [_]
                      tunnel: w718 -> [w726]
                      tunnel: [w725] -> w717
                      n388 = call "Drive Straight.vi"("Angle robot facing"=-90.0) -> ("Arcade drive x"=w723:dbl)  [unwired: 9 in, 1 out]
                      n389 = Wait (ms)(milliseconds to wait=u32 50) -> ()  [unwired: 1 out]
                      n390 = call-poly <vilib>:"WPI_RobotDriveArcadeDrive.vi"("Y axis value"=-0.65, "X axis value"=w723, "RobotDriveDevRef"=w726) -> ("RobotDriveDevRef"=w725:T6)  [unwired: 6 in, 2 out]
                    }
                  }
                }
                n391 = call "Turn To Angle.vi"(7:w682, "Speed/Direction"=-0.7, "Angle"=-115.0) -> ("drive.lvclass"=w674:refnum<class "drive.lvclass">)  [unwired: 8 in]
                n392 = disable-structure shown="Enabled" {
                  disable-tunnel: w674 -> [w731 _]
                  frame Disabled {
                    n393 = call "Set Arm Position.vi"("RobotDriveDevRef 2"=w731, "Speed"=0.9, "Setpoint"=620.0) -> ()  [unwired: 8 in, 1 out]
                  }
                  frame Enabled {
                  }
                }
                n394 = call <vilib>:"WPI_MotorControlRefNum Registry Get.vi"("refnum name"="intakeWheels") -> ("MotorControlDevRef"=w692:T7)  [unwired: 9 in, 1 out]
                n395 = for {
                  N: 20 -> [_]
                  tunnel: w692 -> [w739]
                  tunnel: w680 -> [_]
                  n396 = Wait (ms)(milliseconds to wait=u32 50) -> ()  [unwired: 1 out]
                  n397 = call <vilib>:"WPI_MotorControlSetOutput.vi"("Output"=-1.0, "MotorControlDevRef"=w739) -> ()  [unwired: 7 in, 3 out]
                }
              }
              frame 5 {
                # "may be too much"
                # "Defense position 5"
                # "This ensures that the intake wheels spit out the boulder with one second left in auto, no matter if the other\nactions (the last turning part is our real concern) finish."
                # "Lower arm"
                # "Shoot"
                n398 = disable-structure shown="Disabled" {
                  disable-tunnel: w786 -> [w844 _]
                  frame Disabled {
                    n399 = call "Set Arm Position.vi"("RobotDriveDevRef 2"=w844, "Speed"=0.8, "Setpoint"=480.0) -> ()  [unwired: 8 in, 1 out]
                  }
                  frame Enabled {
                  }
                }
                n400 = call <vilib>:"WPI_AccelerometerRefNum Registry Get.vi"("refnum name"="accel") -> ("AccelerometerDevRef"=w791:T17)  [unwired: 9 in, 1 out]
                n401 = while {
                  tunnel: w777 -> [w818]
                  tunnel: [w817] -> w776
                  stop <- w817 stop-if-true
                  n402 = call "Timeout.vi"("Start Time In"=w818, "Time Limit"=u32 14000) -> ("Timeout"=w817:bool)  [unwired: 8 in, 1 out]
                  n403 = Wait (ms)(milliseconds to wait=u32 300) -> ()  [unwired: 1 out]
                }
                n404 = Tick Count (ms)() -> (millisecond timer value=w783:u32)
                n405 = while {
                  tunnel: w791 -> [w864]
                  tunnel: w786 -> [w856]
                  tunnel: [w855] -> w780
                  tunnel: [w854] -> _
                  tunnel: w783 -> [w851]
                  stop <- w853 stop-if-true
                  n406 = disable-structure shown="Enabled" {
                    disable-tunnel: [w867 0.0 ("X axis value")] -> w849
                    disable-tunnel: [u32 10000 ("Time Limit") u32 10000 ("Time Limit")] -> w848
                    frame Enabled {
                      n407 = call "Drive Straight.vi"("Angle robot facing"=1.0) -> ("Arcade drive x"=w867:dbl)  [unwired: 9 in, 1 out]
                    }
                    frame Disabled {
                    }
                  }
                  n408 = call <vilib>:"WPI_AccelerometerGetAcceleration.vi"("AccelerometerDevRef"=w864) -> ("Accelerations"=w863:T23, "AccelerometerDevRef"=w854:T17)  [unwired: 8 in, 1 out]
                  n409 = call "Timeout.vi"("Start Time In"=w851, "Time Limit"=w848) -> ("Timeout"=w850:bool)  [unwired: 8 in, 1 out]
                  n410 = Unbundle By Name(w863) -> ("Y-Axis"=w859:dbl)
                  n411 = In Range and Coerce(upper limit=0.8, x=w859, lower limit=-0.8) -> (In Range?=w860:bool)  [unwired: 1 out]
                  n412 = Not(x=w860) -> (.not. x?=w852:bool)
                  n413 = call-poly <vilib>:"WPI_RobotDriveArcadeDrive.vi"("Y axis value"=-0.65, "X axis value"=w849, "RobotDriveDevRef"=w856) -> ("RobotDriveDevRef"=w855:T6)  [unwired: 6 in, 2 out]
                  n414 = Or(x=w852, y=w850) -> (x .or. y?=w853:bool)
                  n415 = Wait (ms)(milliseconds to wait=u32 20) -> ()  [unwired: 1 out]
                }
                n416 = disable-structure shown="Disabled" {
                  frame Disabled {
                    n417 = call "Turn And Shoot.vi"("Turning Angle"=-95.0) -> ()  [unwired: 11 in]
                  }
                  frame Enabled {
                  }
                }
                n418 = for {
                  N: 1 -> [_]
                  tunnel: [w837] -> w779
                  tunnel: w780 -> [w837]
                  n419 = Wait (ms)(milliseconds to wait=u32 350) -> ()  [unwired: 1 out]
                }
                n420 = call <vilib>:"WPI_RobotDriveRefNum Registry Get.vi"("refnum name"="intakeDevice") -> ("RobotDriveDevRef"=w770:T6)  [unwired: 9 in, 1 out]
                n421 = call <vilib>:"WPI_SwitchRefNum Registry Get.vi"("refnum name"="mechanismSwitch") -> ("SwitchDevRef"=w766:T14)  [unwired: 9 in, 1 out]
                n422 = call <vilib>:"WPI_GyroRefNum Registry Get.vi"("refnum name"="Gyro") -> ("GyroDevRef"=w763:T2)  [unwired: 9 in, 1 out]
                n423 = call "Forward For inch.vi"("Angle"=0.0 ("Angle robot facing"), "Speed"=0.6, "Distance"=-6.0, "drive.lvclass"=w779) -> ("drive.lvclass"=w768:refnum<class "drive.lvclass">)  [unwired: 7 in]
                n424 = for {
                  N: 175 -> [_]
                  tunnel: w770 -> [w813]
                  tunnel: w768 -> [_]
                  tunnel: [w811] -> _
                  tunnel: w766 -> [w809]
                  stop <- w810 stop-if-true
                  n425 = call <vilib>:"WPI_SwitchGetLimitValue.vi"("SwitchDevRef"=w809) -> ("Switch Pressed"=w810:bool)  [unwired: 8 in, 2 out]
                  n426 = call-poly <vilib>:"WPI_RobotDriveArcadeDrive.vi"("Y axis value"=-0.7, "X axis value"=0.0, "RobotDriveDevRef"=w813) -> ("RobotDriveDevRef"=w811:T6)  [unwired: 6 in, 2 out]
                  n427 = Wait (ms)(milliseconds to wait=u32 20) -> ()  [unwired: 1 out]
                }
                n428 = disable-structure shown="Enabled" {
                  disable-tunnel: w768 -> [w794 w799]
                  disable-tunnel: [w793 w798] -> w765
                  disable-tunnel: w763 -> [_ w797]
                  frame Disabled {
                    n429 = call "Turn To Angle.vi"(7:w794, "Speed/Direction"=-1.0, "Angle"=-70.0) -> ("drive.lvclass"=w793:refnum<class "drive.lvclass">)  [unwired: 8 in]
                  }
                  frame Enabled {
                    n430 = while {
                      tunnel: w799 -> [w808]
                      tunnel: [w807] -> w798
                      tunnel: w797 -> [w804]
                      stop <- w801 stop-if-true
                      n431 = call <vilib>:"WPI_GyroGetAngle.vi"("GyroDevRef"=w804) -> ("Angle"=w803:dbl)  [unwired: 6 in, 4 out]
                      n432 = Wait (ms)(milliseconds to wait=u32 30) -> ()  [unwired: 1 out]
                      n433 = call-poly <vilib>:"WPI_RobotDriveArcadeDrive.vi"("Y axis value"=0.0, "X axis value"=-1.0, "RobotDriveDevRef"=w808) -> ("RobotDriveDevRef"=w807:T6)  [unwired: 6 in, 2 out]
                      n434 = Less Or Equal?(x=w803, y=-70.0) -> (x <= y?=w801:bool)
                    }
                  }
                }
                n435 = call-poly <vilib>:"NT Write Value.vi"("Numeric"=3.0, "Name"="Template") -> ()  [unwired: 9 in, 1 out]
                n436 = disable-structure shown="Enabled" {
                  disable-tunnel: w765 -> [w821 w826]
                  disable-tunnel: [w820 w825] -> w778
                  frame Disabled {
                    n437 = call "Forward For inch.vi"("Angle"=-90.0 ("Angle robot facing"), "Speed"=-0.6, "Distance"=72.0, "drive.lvclass"=w821) -> ("drive.lvclass"=w820:refnum<class "drive.lvclass">)  [unwired: 7 in]
                  }
                  frame Enabled {
                    n438 = disable-structure shown="Disabled" {
                      disable-tunnel: w826 -> [w830 _]
                      frame Disabled {
                        n439 = call "Set Arm Position.vi"("RobotDriveDevRef 2"=w830, "Speed"=0.8, "Setpoint"=550.0) -> ()  [unwired: 8 in, 1 out]
                      }
                      frame Enabled {
                      }
                    }
                    n440 = for {
                      N: 20 -> [_]
                      tunnel: w826 -> [w834]
                      tunnel: [w833] -> w825
                      n441 = call "Drive Straight.vi"("Angle robot facing"=-80.0) -> ("Arcade drive x"=w831:dbl)  [unwired: 9 in, 1 out]
                      n442 = Wait (ms)(milliseconds to wait=u32 50) -> ()  [unwired: 1 out]
                      n443 = call-poly <vilib>:"WPI_RobotDriveArcadeDrive.vi"("Y axis value"=-0.55, "X axis value"=w831, "RobotDriveDevRef"=w834) -> ("RobotDriveDevRef"=w833:T6)  [unwired: 6 in, 2 out]
                    }
                  }
                }
                n444 = call "Turn To Angle.vi"(7:w778, "Speed/Direction"=0.7, "Angle"=-65.0) -> ("drive.lvclass"=w772:refnum<class "drive.lvclass">)  [unwired: 8 in]
                n445 = disable-structure shown="Enabled" {
                  disable-tunnel: w772 -> [w839 _]
                  frame Disabled {
                    n446 = call "Set Arm Position.vi"("RobotDriveDevRef 2"=w839, "Speed"=0.9, "Setpoint"=620.0) -> ()  [unwired: 8 in, 1 out]
                  }
                  frame Enabled {
                  }
                }
                n447 = call <vilib>:"WPI_MotorControlRefNum Registry Get.vi"("refnum name"="intakeWheels") -> ("MotorControlDevRef"=w788:T7)  [unwired: 9 in, 1 out]
                n448 = for {
                  N: 20 -> [_]
                  tunnel: w788 -> [w847]
                  tunnel: w776 -> [_]
                  tunnel: w765 -> [_]
                  n449 = Wait (ms)(milliseconds to wait=u32 50) -> ()  [unwired: 1 out]
                  n450 = call <vilib>:"WPI_MotorControlSetOutput.vi"("Output"=-1.0, "MotorControlDevRef"=w847) -> ()  [unwired: 7 in, 3 out]
                }
              }
              frame 4 {
                w882 = 75.0 ("Angle")
                # "may be too much"
                # "Turn and align as if coming out\nof defense 5"
                # "Defense position 4"
                # "disabled case for driving to wall\n at an angle"
                # "Raise arm so it doesn't\ndrag on ground"
                # "This ensures that the intake wheels spit out the boulder with one second left in auto, no matter if the other\nactions (the last turning part is our real concern) finish."
                # "Lower arm"
                # "Shoot"
                n451 = disable-structure shown="Disabled" {
                  disable-tunnel: w887 -> [w946 _]
                  frame Disabled {
                    n452 = call "Set Arm Position.vi"("RobotDriveDevRef 2"=w946, "Speed"=0.8, "Setpoint"=480.0) -> ()  [unwired: 8 in, 1 out]
                  }
                  frame Enabled {
                  }
                }
                n453 = call "Turn To Angle.vi"(7:w887, "Speed/Direction"=0.75, "Angle"=w882) -> ("drive.lvclass"=w889:refnum<class "drive.lvclass">)  [unwired: 8 in]
                n454 = call "Forward For inch.vi"("Angle"=w882, "Speed"=-0.7, "Distance"=51.0, "drive.lvclass"=w889) -> ("drive.lvclass"=w888:refnum<class "drive.lvclass">)  [unwired: 7 in]
                n455 = call <vilib>:"WPI_AccelerometerRefNum Registry Get.vi"("refnum name"="accel") -> ("AccelerometerDevRef"=w907:T17)  [unwired: 9 in, 1 out]
                n456 = while {
                  tunnel: w897 -> [w922]
                  tunnel: [w921] -> w896
                  stop <- w921 stop-if-true
                  n457 = call "Timeout.vi"("Start Time In"=w922, "Time Limit"=u32 14000) -> ("Timeout"=w921:bool)  [unwired: 8 in, 1 out]
                  n458 = Wait (ms)(milliseconds to wait=u32 300) -> ()  [unwired: 1 out]
                }
                n459 = Tick Count (ms)() -> (millisecond timer value=w900:u32)
                n460 = call "Turn To Angle.vi"(7:w888, "Speed/Direction"=-0.75, "Angle"=0.0) -> ("drive.lvclass"=w886:refnum<class "drive.lvclass">)  [unwired: 8 in]
                n461 = while {
                  tunnel: w907 -> [w966]
                  tunnel: w886 -> [w958]
                  tunnel: [w957] -> w872
                  tunnel: [w956] -> _
                  tunnel: w900 -> [w953]
                  stop <- w955 stop-if-true
                  n462 = disable-structure shown="Enabled" {
                    disable-tunnel: [w969 0.0 ("X axis value")] -> w951
                    disable-tunnel: [u32 15000 ("Time Limit") u32 10000 ("Time Limit")] -> w950
                    frame Enabled {
                      n463 = call "Drive Straight.vi"("Angle robot facing"=3.0) -> ("Arcade drive x"=w969:dbl)  [unwired: 9 in, 1 out]
                    }
                    frame Disabled {
                    }
                  }
                  n464 = call <vilib>:"WPI_AccelerometerGetAcceleration.vi"("AccelerometerDevRef"=w966) -> ("Accelerations"=w965:T23, "AccelerometerDevRef"=w956:T17)  [unwired: 8 in, 1 out]
                  n465 = call "Timeout.vi"("Start Time In"=w953, "Time Limit"=w950) -> ("Timeout"=w952:bool)  [unwired: 8 in, 1 out]
                  n466 = Unbundle By Name(w965) -> ("Y-Axis"=w961:dbl)
                  n467 = In Range and Coerce(upper limit=0.8, x=w961, lower limit=-0.8) -> (In Range?=w962:bool)  [unwired: 1 out]
                  n468 = Not(x=w962) -> (.not. x?=w954:bool)
                  n469 = call-poly <vilib>:"WPI_RobotDriveArcadeDrive.vi"("Y axis value"=-0.65, "X axis value"=w951, "RobotDriveDevRef"=w958) -> ("RobotDriveDevRef"=w957:T6)  [unwired: 6 in, 2 out]
                  n470 = Or(x=w954, y=w952) -> (x .or. y?=w955:bool)
                  n471 = Wait (ms)(milliseconds to wait=u32 20) -> ()  [unwired: 1 out]
                }
                n472 = disable-structure shown="Disabled" {
                  frame Disabled {
                    n473 = call "Turn And Shoot.vi"("Turning Angle"=-95.0) -> ()  [unwired: 11 in]
                  }
                  frame Enabled {
                  }
                }
                n474 = flat-sequence {
                  tunnel: w872 -> [w910]
                  tunnel: [w910] -> w871
                  frame #0 {
                    n475 = Wait (ms)(milliseconds to wait=u32 350 ("time (ms)")) -> ()  [unwired: 1 out]
                  }
                }
                n476 = call <vilib>:"WPI_RobotDriveRefNum Registry Get.vi"("refnum name"="intakeDevice") -> ("RobotDriveDevRef"=w878:T6)  [unwired: 9 in, 1 out]
                n477 = call <vilib>:"WPI_SwitchRefNum Registry Get.vi"("refnum name"="mechanismSwitch") -> ("SwitchDevRef"=w875:T14)  [unwired: 9 in, 1 out]
                n478 = call "Forward For inch.vi"("Angle"=0.0 ("Angle robot facing"), "Speed"=0.6, "Distance"=-6.0, "drive.lvclass"=w871) -> ("drive.lvclass"=w874:refnum<class "drive.lvclass">)  [unwired: 7 in]
                n479 = for {
                  N: 175 -> [_]
                  tunnel: w878 -> [w915]
                  tunnel: [w913] -> _
                  tunnel: w875 -> [w911]
                  tunnel: w874 -> [_]
                  stop <- w912 stop-if-true
                  n480 = call <vilib>:"WPI_SwitchGetLimitValue.vi"("SwitchDevRef"=w911) -> ("Switch Pressed"=w912:bool)  [unwired: 8 in, 2 out]
                  n481 = call-poly <vilib>:"WPI_RobotDriveArcadeDrive.vi"("Y axis value"=-0.7, "X axis value"=0.0, "RobotDriveDevRef"=w915) -> ("RobotDriveDevRef"=w913:T6)  [unwired: 6 in, 2 out]
                  n482 = Wait (ms)(milliseconds to wait=u32 20) -> ()  [unwired: 1 out]
                }
                n483 = disable-structure shown="Enabled" {
                  disable-tunnel: [-100.0 ("Angle") -70.0 ("Angle")] -> w891
                  frame Disabled {
                  }
                  frame Enabled {
                  }
                }
                n484 = call "Turn To Angle.vi"(7:w874, "Speed/Direction"=-0.95, "Angle"=w891) -> ("drive.lvclass"=w873:refnum<class "drive.lvclass">)  [unwired: 8 in]
                n485 = call-poly <vilib>:"NT Write Value.vi"("Numeric"=3.0, "Name"="Template") -> ()  [unwired: 9 in, 1 out]
                n486 = disable-structure shown="Enabled" {
                  disable-tunnel: w873 -> [w925 w930]
                  disable-tunnel: [w924 w929] -> w898
                  frame Disabled {
                    n487 = call "Forward For inch.vi"("Angle"=-90.0 ("Angle robot facing"), "Speed"=-0.6, "Distance"=72.0, "drive.lvclass"=w925) -> ("drive.lvclass"=w924:refnum<class "drive.lvclass">)  [unwired: 7 in]
                  }
                  frame Enabled {
                    n488 = disable-structure shown="Disabled" {
                      disable-tunnel: w930 -> [w934 _]
                      frame Disabled {
                        n489 = call "Set Arm Position.vi"("RobotDriveDevRef 2"=w934, "Speed"=0.8, "Setpoint"=550.0) -> ()  [unwired: 8 in, 1 out]
                      }
                      frame Enabled {
                      }
                    }
                    n490 = for {
                      N: 20 -> [_]
                      tunnel: w930 -> [w938]
                      tunnel: [w937] -> w929
                      n491 = call "Drive Straight.vi"("Angle robot facing"=-80.0) -> ("Arcade drive x"=w935:dbl)  [unwired: 9 in, 1 out]
                      n492 = Wait (ms)(milliseconds to wait=u32 50) -> ()  [unwired: 1 out]
                      n493 = call-poly <vilib>:"WPI_RobotDriveArcadeDrive.vi"("Y axis value"=-0.55, "X axis value"=w935, "RobotDriveDevRef"=w938) -> ("RobotDriveDevRef"=w937:T6)  [unwired: 6 in, 2 out]
                    }
                  }
                }
                n494 = call "Turn To Angle.vi"(7:w898, "Speed/Direction"=0.7, "Angle"=-65.0) -> ("drive.lvclass"=w890:refnum<class "drive.lvclass">)  [unwired: 8 in]
                n495 = disable-structure shown="Enabled" {
                  disable-tunnel: w890 -> [w941 _]
                  frame Disabled {
                    n496 = call "Set Arm Position.vi"("RobotDriveDevRef 2"=w941, "Speed"=0.9, "Setpoint"=620.0) -> ()  [unwired: 8 in, 1 out]
                  }
                  frame Enabled {
                  }
                }
                n497 = call <vilib>:"WPI_MotorControlRefNum Registry Get.vi"("refnum name"="intakeWheels") -> ("MotorControlDevRef"=w904:T7)  [unwired: 9 in, 1 out]
                n498 = for {
                  N: 20 -> [_]
                  tunnel: w904 -> [w949]
                  tunnel: w896 -> [_]
                  tunnel: w873 -> [_]
                  n499 = Wait (ms)(milliseconds to wait=u32 50) -> ()  [unwired: 1 out]
                  n500 = call <vilib>:"WPI_MotorControlSetOutput.vi"("Output"=-1.0, "MotorControlDevRef"=w949) -> ()  [unwired: 7 in, 3 out]
                }
              }
              frame 2 {
                (unwired) 140.0 ("Camera Angle Vertical")
                (unwired) 145.0 ("Camera Angle")
                w984 = -60.0 ("Angle")
                n501 = call "Set Arm Position.vi"("RobotDriveDevRef 2"=w975, "Setpoint"=350.0) -> ()  [unwired: 9 in, 1 out]
                n502 = call "Turn To Angle.vi"(7:w975, "Speed/Direction"=-0.6, "Angle"=w984) -> ("drive.lvclass"=w988:refnum<class "drive.lvclass">)  [unwired: 8 in]
                n503 = call "Forward For inch.vi"("Angle"=w984, "Speed"=-0.6, "Distance"=56.0, "drive.lvclass"=w988) -> ("drive.lvclass"=w983:refnum<class "drive.lvclass">)  [unwired: 7 in]
                n504 = call "Turn To Angle.vi"(7:w983, "Speed/Direction"=0.6, "Angle"=0.0) -> ("drive.lvclass"=w977:refnum<class "drive.lvclass">)  [unwired: 8 in]
                n505 = call "Set Arm Position.vi"("RobotDriveDevRef 2"=w977, "Speed"=0.8, "Setpoint"=550.0) -> ()  [unwired: 8 in, 1 out]
                n506 = call "Auto Aim.vi"("Turning Angle"=40.0, "RobotDriveDevRef in"=w977, "Angle robot facing"=0.0, "Target Boundries"=cluster{"Upper":dbl, "Lower":dbl} {"Upper"=85.0, "Lower"=78.0}) -> ()  [unwired: 8 in]
              }
              frame 3 {
                w1000 = 80.0 ("Angle")
                # "NEXT TIME MAKE SUBVI FOR THESE SHARED ACTIONS"
                # "may be too much"
                # "Turn and align as if coming out\nof defense 5"
                # "Defense position 3"
                # "disabled case for driving to wall\n at an angle"
                # "Raise arm so it doesn't\ndrag on ground"
                # "This ensures that the intake wheels spit out the boulder with one second left in auto, no matter if the other\nactions (the last turning part is our real concern) finish."
                # "Lower arm"
                # "Shoot"
                n507 = call "Turn To Angle.vi"(7:w989, "Speed/Direction"=0.75, "Angle"=w1000) -> ("drive.lvclass"=w1006:refnum<class "drive.lvclass">)  [unwired: 8 in]
                n508 = call "Forward For inch.vi"("Angle"=w1000, "Speed"=-0.75, "Distance"=102.0, "drive.lvclass"=w1006) -> ("drive.lvclass"=w1005:refnum<class "drive.lvclass">)  [unwired: 7 in]
                n509 = call <vilib>:"WPI_AccelerometerRefNum Registry Get.vi"("refnum name"="accel") -> ("AccelerometerDevRef"=w1026:T17)  [unwired: 9 in, 1 out]
                n510 = while {
                  tunnel: w990 -> [w1039]
                  tunnel: [w1038] -> w1013
                  stop <- w1038 stop-if-true
                  n511 = call "Timeout.vi"("Start Time In"=w1039, "Time Limit"=u32 14000) -> ("Timeout"=w1038:bool)  [unwired: 8 in, 1 out]
                  n512 = Wait (ms)(milliseconds to wait=u32 300) -> ()  [unwired: 1 out]
                }
                n513 = Tick Count (ms)() -> (millisecond timer value=w1019:u32)
                n514 = call "Turn To Angle.vi"(7:w1005, "Speed/Direction"=-0.75, "Angle"=0.0) -> ("drive.lvclass"=w1004:refnum<class "drive.lvclass">)  [unwired: 8 in]
                n515 = while {
                  tunnel: w1026 -> [w1082]
                  tunnel: w1004 -> [w1074]
                  tunnel: [w1073] -> w1016
                  tunnel: [w1072] -> _
                  tunnel: w1019 -> [w1069]
                  stop <- w1071 stop-if-true
                  n516 = disable-structure shown="Enabled" {
                    disable-tunnel: [w1085 0.0 ("X axis value")] -> w1067
                    disable-tunnel: [u32 10000 ("Time Limit") u32 10000 ("Time Limit")] -> w1066
                    frame Enabled {
                      n517 = call "Drive Straight.vi"("Angle robot facing"=3.0) -> ("Arcade drive x"=w1085:dbl)  [unwired: 9 in, 1 out]
                    }
                    frame Disabled {
                    }
                  }
                  n518 = call <vilib>:"WPI_AccelerometerGetAcceleration.vi"("AccelerometerDevRef"=w1082) -> ("Accelerations"=w1081:T23, "AccelerometerDevRef"=w1072:T17)  [unwired: 8 in, 1 out]
                  n519 = call "Timeout.vi"("Start Time In"=w1069, "Time Limit"=w1066) -> ("Timeout"=w1068:bool)  [unwired: 8 in, 1 out]
                  n520 = Unbundle By Name(w1081) -> ("Y-Axis"=w1077:dbl)
                  n521 = In Range and Coerce(upper limit=0.8, x=w1077, lower limit=-0.8) -> (In Range?=w1078:bool)  [unwired: 1 out]
                  n522 = Not(x=w1078) -> (.not. x?=w1070:bool)
                  n523 = call-poly <vilib>:"WPI_RobotDriveArcadeDrive.vi"("Y axis value"=-0.65, "X axis value"=w1067, "RobotDriveDevRef"=w1074) -> ("RobotDriveDevRef"=w1073:T6)  [unwired: 6 in, 2 out]
                  n524 = Or(x=w1070, y=w1068) -> (x .or. y?=w1071:bool)
                  n525 = Wait (ms)(milliseconds to wait=u32 20) -> ()  [unwired: 1 out]
                }
                n526 = disable-structure shown="Disabled" {
                  frame Disabled {
                    n527 = call "Turn And Shoot.vi"("Turning Angle"=-95.0) -> ()  [unwired: 11 in]
                  }
                  frame Enabled {
                  }
                }
                n528 = for {
                  N: 1 -> [_]
                  tunnel: [w1058] -> w1015
                  tunnel: w1016 -> [w1058]
                  n529 = Wait (ms)(milliseconds to wait=u32 350) -> ()  [unwired: 1 out]
                }
                n530 = call <vilib>:"WPI_RobotDriveRefNum Registry Get.vi"("refnum name"="intakeDevice") -> ("RobotDriveDevRef"=w996:T6)  [unwired: 9 in, 1 out]
                n531 = call <vilib>:"WPI_SwitchRefNum Registry Get.vi"("refnum name"="mechanismSwitch") -> ("SwitchDevRef"=w993:T14)  [unwired: 9 in, 1 out]
                n532 = call "Forward For inch.vi"("Angle"=0.0 ("Angle robot facing"), "Speed"=0.6, "Distance"=-6.0, "drive.lvclass"=w1015) -> ("drive.lvclass"=w992:refnum<class "drive.lvclass">)  [unwired: 7 in]
                n533 = for {
                  N: 175 -> [_]
                  tunnel: w996 -> [w1032]
                  tunnel: [w1030] -> _
                  tunnel: w993 -> [w1028]
                  tunnel: w992 -> [_]
                  stop <- w1029 stop-if-true
                  n534 = call <vilib>:"WPI_SwitchGetLimitValue.vi"("SwitchDevRef"=w1028) -> ("Switch Pressed"=w1029:bool)  [unwired: 8 in, 2 out]
                  n535 = call-poly <vilib>:"WPI_RobotDriveArcadeDrive.vi"("Y axis value"=-0.6, "X axis value"=0.0, "RobotDriveDevRef"=w1032) -> ("RobotDriveDevRef"=w1030:T6)  [unwired: 6 in, 2 out]
                  n536 = Wait (ms)(milliseconds to wait=u32 20) -> ()  [unwired: 1 out]
                }
                n537 = disable-structure shown="Enabled" {
                  disable-tunnel: [-100.0 ("Angle") -70.0 ("Angle")] -> w1008
                  frame Disabled {
                  }
                  frame Enabled {
                  }
                }
                n538 = call "Turn To Angle.vi"(7:w992, "Speed/Direction"=-0.9, "Angle"=w1008) -> ("drive.lvclass"=w991:refnum<class "drive.lvclass">)  [unwired: 8 in]
                n539 = call-poly <vilib>:"NT Write Value.vi"("Numeric"=3.0, "Name"="Template") -> ()  [unwired: 9 in, 1 out]
                n540 = disable-structure shown="Enabled" {
                  disable-tunnel: w991 -> [w1042 w1047]
                  disable-tunnel: [w1041 w1046] -> w1014
                  frame Disabled {
                    n541 = call "Forward For inch.vi"("Angle"=-90.0 ("Angle robot facing"), "Speed"=-0.6, "Distance"=72.0, "drive.lvclass"=w1042) -> ("drive.lvclass"=w1041:refnum<class "drive.lvclass">)  [unwired: 7 in]
                  }
                  frame Enabled {
                    n542 = disable-structure shown="Disabled" {
                      disable-tunnel: w1047 -> [w1051 _]
                      frame Disabled {
                        n543 = call "Set Arm Position.vi"("RobotDriveDevRef 2"=w1051, "Speed"=0.8, "Setpoint"=550.0) -> ()  [unwired: 8 in, 1 out]
                      }
                      frame Enabled {
                      }
                    }
                    n544 = for {
                      N: 20 -> [_]
                      tunnel: w1047 -> [w1055]
                      tunnel: [w1054] -> w1046
                      n545 = call "Drive Straight.vi"("Angle robot facing"=-80.0) -> ("Arcade drive x"=w1052:dbl)  [unwired: 9 in, 1 out]
                      n546 = Wait (ms)(milliseconds to wait=u32 50) -> ()  [unwired: 1 out]
                      n547 = call-poly <vilib>:"WPI_RobotDriveArcadeDrive.vi"("Y axis value"=-0.55, "X axis value"=w1052, "RobotDriveDevRef"=w1055) -> ("RobotDriveDevRef"=w1054:T6)  [unwired: 6 in, 2 out]
                    }
                  }
                }
                n548 = call "Turn To Angle.vi"(7:w1014, "Speed/Direction"=0.7, "Angle"=-65.0) -> ("drive.lvclass"=w1007:refnum<class "drive.lvclass">)  [unwired: 8 in]
                n549 = disable-structure shown="Enabled" {
                  disable-tunnel: w1007 -> [w1060 _]
                  frame Disabled {
                    n550 = call "Set Arm Position.vi"("RobotDriveDevRef 2"=w1060, "Speed"=0.9, "Setpoint"=620.0) -> ()  [unwired: 8 in, 1 out]
                  }
                  frame Enabled {
                  }
                }
                n551 = call <vilib>:"WPI_MotorControlRefNum Registry Get.vi"("refnum name"="intakeWheels") -> ("MotorControlDevRef"=w1023:T7)  [unwired: 9 in, 1 out]
                n552 = for {
                  N: 20 -> [_]
                  tunnel: w1023 -> [w1065]
                  tunnel: w1013 -> [_]
                  tunnel: w991 -> [_]
                  n553 = Wait (ms)(milliseconds to wait=u32 50) -> ()  [unwired: 1 out]
                  n554 = call <vilib>:"WPI_MotorControlSetOutput.vi"("Output"=-1.0, "MotorControlDevRef"=w1065) -> ()  [unwired: 7 in, 3 out]
                }
              }
            }
            n555 = call-poly <vilib>:"NT Write Value.vi"("Numeric"=w663, "Name"="Template") -> ()  [unwired: 9 in, 1 out]
          }
        }
        n556 = disable-structure shown="Disabled" {
          frame Disabled {
            # "This slowly pulls the ball in so it doesn't fall out"
            n557 = while {
              stop <- w240 stop-if-true
              n558 = Wait (ms)(milliseconds to wait=u32 50) -> ()  [unwired: 1 out]
              n559 = local read "Stop Wheel Loop"() -> (w240:bool)
              n560 = call <vilib>:"WPI_MotorControlRefNum Registry Get.vi"("refnum name"="intakeWheels") -> ("MotorControlDevRef"=w242:T7)  [unwired: 9 in, 1 out]
              n561 = call <vilib>:"WPI_MotorControlSetOutput.vi"("Output"=0.4, "MotorControlDevRef"=w242) -> ()  [unwired: 7 in, 3 out]
            }
          }
          frame Enabled {
          }
        }
        "Stop Wheel Loop" <- FALSE
      }
      frame 2 {
        # "Shoot here"
        n562 = call <vilib>:"WPI_RobotDriveRefNum Registry Get.vi"("refnum name"="Drive 1") -> ("RobotDriveDevRef"=w1099:T6)  [unwired: 9 in, 1 out]
        n563 = call "Set Arm Position.vi"("RobotDriveDevRef 2"=w1099, "Speed"=0.8, "Setpoint"=550.0) -> ()  [unwired: 8 in, 1 out]
        n564 = call "Forward For inch.vi"("Angle"=0.0 ("Angle robot facing"), "Speed"=-0.65, "Distance"=90.0, "drive.lvclass"=w1099) -> ("drive.lvclass"=w1090:refnum<class "drive.lvclass">)  [unwired: 7 in]
        n565 = call-poly <vilib>:"NT Write Value.vi"("Numeric"=3.0, "Name"="Template") -> ()  [unwired: 9 in, 1 out]
        n566 = call <vilib>:"WPI_MotorControlRefNum Registry Get.vi"("refnum name"="intakeWheels") -> ("error out"=w1091:errorcluster, "MotorControlDevRef"=w1092:T7)  [unwired: 9 in]
        n567 = for {
          N: 20 -> [_]
          tunnel: w1091 -> [w1107]
          tunnel: w1092 -> [w1106]
          tunnel: w1090 -> [_]
          n568 = Wait (ms)(milliseconds to wait=u32 50) -> ()  [unwired: 1 out]
          n569 = call <vilib>:"WPI_MotorControlSetOutput.vi"("error in (no error)"=w1107, "Output"=-1.0, "MotorControlDevRef"=w1106) -> ()  [unwired: 6 in, 3 out]
        }
      }
    }
  }
